vi "Q14070-Z060B bak.vi"() -> ()   [LabVIEW 2013]
uses:
  <vilib>/Utility/file.llb/Read From Spreadsheet File (string).vi
  <vilib>/express/express arith-compare/Formula/XNode/ExpressFormulaBlockNode.xnode
  PCI8622_32.dll
  <vilib>/printing/EasyPrintingControls.llb/contents.ctl
  <vilib>/Utility/NIReport.llb/NI_ReportGenerationCore.lvlib
  <vilib>/printing/EasyPrintingControls.llb/report_type.ctl
  <vilib>/printing/EasyPrinting.llb/Easy Print VI Panel or Documentation (path).vi
  <vilib>/Utility/NIReport.llb/NI_report.lvclass
panel:
  out "最大轴向力标准(N)":dbl=200.0 caption="L+Lmax(mm)" format="%#.3f"
  out "右平均轴向力(N)":dbl caption="L+Lmax(mm)" format="%#.3f"
  out "左平均轴向力(N)":dbl caption="最大位移偏离Lmax(mm)" format="%#.3f"
  in  "确定按钮":bool
  out "员工ID":string
  in  "出支线工步号":dbl
  out "报警提示":string
  in  "报警工步号":dbl
  out "急停":bool
  in  "机械间隙值":dbl
  out "DeviceHandle":u32
  in  "轴向力设定次数":dbl=5.0
  in  "最小间隙(mm)":dbl=0.0005 format="%#.3f"
  out "本备料状态H":bool
  out "本测试状态H":bool
  out "本自动状态H":bool
  out "夹头松开":bool
  out "测头右位":bool
  out "测头左位":bool
  in  "测头气缸右移":bool
  in  "测头气缸左移":bool
  in  "轴向力已做次数":dbl
  out "轴向力及全行程间隙合格":bool
  out "轴向力启动":bool
  out "间隙启动":bool
  out "夹头夹紧位":bool
  in  "夹头松开":bool
  in  "夹头夹紧":bool
  out "找帽扭矩":dbl=1.0 caption="压力传感器" format="%#.2f"
  out "error out":errorcluster
  out "型号数量":i32
  out "error out 4":errorcluster
  in  "间隙设定调整次数":dbl=5.0
  out "读取产品ID":string
  out "本备料状态":bool
  out "本测试状态":bool
  out "本自动状态":bool
  out "FGCS":string
  out "KSJJ":string
  out "Z060BRFID":string
  out "轴向力Y":dbl[](array[numeric])
  out "轴向力X":dbl[](array[numeric])
  out "间隙X数组":dbl[](array[numeric])
  out "间隙Y数组":dbl[](array[numeric])
  out "error out 3":errorcluster caption="错误输出"
  out "rfid工步号":u32
  out "芯片ID":string="201209190001"
  out "rfid完成":bool
  out "rfid触发":bool
  out "本序已做":bool
  in  "回零完成":bool
  in  "电动缸回零":bool
  in  "单点间隙已调试次数":dbl
  in  "需调整角度(度)":dbl
  in  "转向器中心":dbl
  out "扭矩到达":bool
  out "黄灯":bool
  out "红灯":bool
  out "基准位移":dbl caption="压力传感器" format="%#.4f"
  out "上序不合格":bool
  out "单点间隙合格":bool
  out "上序合格":bool
  out "测头机构电机":u32
  out "复位":bool
  in  "型号选择":u16(ring)=1 items=["J709", "J728", "J706"]
  in  "联线按钮":bool
  in  "工步号":u32
  in  "产品ID":string="201209190001"
  out "间隙位移(mm)":dbl caption="压力传感器" format="%#.3f"
  out "齿条推拉力(N)":dbl format="%#.2f"
  out "齿条扭矩(Nm)":dbl format="%#.2f"
  out "通讯状态":bool
  in  "员工ID":string
  out "员工姓名":string
  out "工步提示":string
  out "ADODB._Connection Out 2":refnum<k7>
  out "旋转齿条电机":u32
  out "电动缸电机":u32
  in  "停止":bool
  in  "参数加载":bool
  in  "选项卡控件":T1(tab)
  in  "180°外全行程间隙标准(mm)":dbl=0.1 format="%#.3f"
  out "扭动曲线":cluster{"Y":dbl[], "Y":dbl[]}[](graph) caption="压球涨堵头1"
  out "中间位置间隙":dbl caption="间隙值L(mm)" format="%#.3f"
  in  "中间位置最大间隙标准(mm)":dbl=0.07 format="%#.3f"
  out "右180°外全行程间隙":dbl caption="正向最大间隙L1(mm)" format="%#.3f"
  out "左180°外全行程间隙":dbl caption="正向最大间隙L1(mm)" format="%#.3f"
  out "右180°内全行程间隙":dbl caption="正向最大间隙L1(mm)" format="%#.3f"
  out "左180°内全行程间隙":dbl caption="正向最大间隙L1(mm)" format="%#.3f"
  in  "180°内全行程间隙标准(mm)":dbl=0.07 format="%#.3f"
  in  "找帽OK":bool
  out "左全行程间隙":dbl caption="正向最大间隙L1(mm)" format="%#.3f"
  out "右全行程间隙":dbl caption="正向最大间隙L1(mm)" format="%#.3f"
  out "总圈数最大值":dbl
  out "总圈数标准":dbl
  out "总行程最大值":dbl
  out "总行程标准(mm)":dbl
  out "力波动标准(N)":dbl=60.0 caption="L+Lmax(mm)" format="%#.3f"
  out "平均轴向力标准(N)":dbl=100.0 caption="L+Lmax(mm)" format="%#.3f"
  out "右轴向力波动(N)":dbl caption="L+Lmax(mm)" format="%_5f"
  out "右最大轴向力(N)":dbl caption="L+Lmax(mm)" format="%_5f"
  out "左轴向力波动(N)":dbl caption="最大位移偏离Lmax(mm)" format="%_5f"
  out "左最大轴向力(N)":dbl caption="最大位移偏离Lmax(mm)" format="%_5f"
  out "行程跳动曲线":cluster{"Y":dbl[], "Y":dbl[]}[](graph) caption="压球涨堵头1"
  out "平均轴向力标准(N) max":dbl=200.0 caption="L+Lmax(mm)" format="%#.3f"
  out "总行程":dbl format="%_5g"
  out "总圈数":dbl format="%_1f"
  in  "不合格品":bool
  in  "扭矩停止值":dbl=16.0
  in  "齿条右极限":dbl=-70.0 caption="压力传感器" format="%#.2f"
  in  "齿条左极限":dbl=-262.0 caption="压力传感器" format="%#.2f"
  in  "齿条移动速度":dbl=5.0 caption="压力传感器" format="%#.2f"
  in  "旋转齿条轴找帽转速":dbl=5.0 caption="压力传感器" format="%#.2f"
  in  "测量点扭矩":dbl=4.0 caption="压力传感器" format="%#.2f"
  in  "旋转齿条轴测量转速":dbl caption="压力传感器" format="%#.2f"
  in  "测头机构轴后退位":dbl=30.0 caption="压力传感器" format="%#.2f"
  in  "测头机构轴待检位":dbl caption="压力传感器" format="%#.2f"
  in  "测头机构轴检测位":dbl caption="压力传感器" format="%#.2f"
  in  "测头机构轴移动速度":dbl caption="压力传感器" format="%#.2f"
  in  "机械间隙值":dbl=1.0
  in  "夹头松开":bool
  in  "夹头夹紧":bool
  in  "测头气缸右移":bool
  in  "测头气缸左移":bool
  in  "支线下降":bool
  in  "支线顶升":bool
  in  "出支线":bool
  in  "进支线":bool
  in  "主线下降":bool
  in  "主线顶升":bool
  in  "下阻挡器放行":bool
  in  "上阻挡器放行":bool
  in  "测头机构轴使能":bool
  in  "测头机构轴后退":bool
  in  "测头机构轴前进":bool
  in  "电动缸速度(mm/s)":dbl=10.0 format="%#.3f"
  out "电动缸位置(mm)":dbl=10000.0 format="%#.3f"
  in  "旋转齿条轴速度(°/s)":dbl=10.0 format="%#.3f"
  out "旋转齿条轴位置(°)":dbl=10000.0 format="%#.3f"
  in  "测头机构轴速度(mm/s)":dbl=10.0 format="%#.3f"
  out "测头机构轴位置(mm)":dbl=10000.0 format="%#.3f"
  in  "旋转齿条轴右转":bool
  in  "旋转齿条轴左转":bool
  in  "旋转齿条轴使能":bool
  in  "电动缸后退":bool
  in  "电动缸使能":bool
  in  "电动缸前进":bool
  in  "齿条扭矩比例偏移":dbl=1.0 format="%#.2f"
  in  "齿条扭矩零点偏移":dbl format="%#.2f"
  in  "齿条推拉力比例偏移":dbl=1.0 format="%#.2f"
  in  "齿条推拉力零点偏移":dbl format="%#.2f"
  in  "间隙位移比例偏移":dbl=1.0 format="%#.2f"
  in  "间隙位移零点偏移":dbl format="%#.2f"
  in  "传感器参数保存":bool
  in  "参数修改":bool
  in  "参数查询":bool
  in  "参数浏览表":string[][](table)
  # "芜湖机械转向器装配线"
  # "间隙及轴向力检测"
  # "Q14070机械转向器装配线"
  # "湖北唯思凌科装备制造有限公司 设计开发 (C)2015"
  # "间隙测量结果"
  # "间隙测量判定值"
  # "≤"
  # "≤"
  # "≤"
  # "轴向力测量结果"
  # "轴向力测量标准"
  # "≥"
  # "≤"
  # "≥"
  # "≤"
  # "≤"
  # "≥"
  # "不得大于20NM"
  # "传感器校验区"
  # "关于传感器校验：\n1、传感器校验需要由具备资质的单位或部门进行校验。\n2、具备权限的用户才能够修改传感器校验参数和试验参数。\n3、修改校验参数方法：先将比例偏移置为1，修改零点偏移，使零点值与校验的传感器一致；然后根据增幅调整比例偏移。"
  # "注意：\n具备权限的用户才能够修改传感器校验参数和试验参数！"
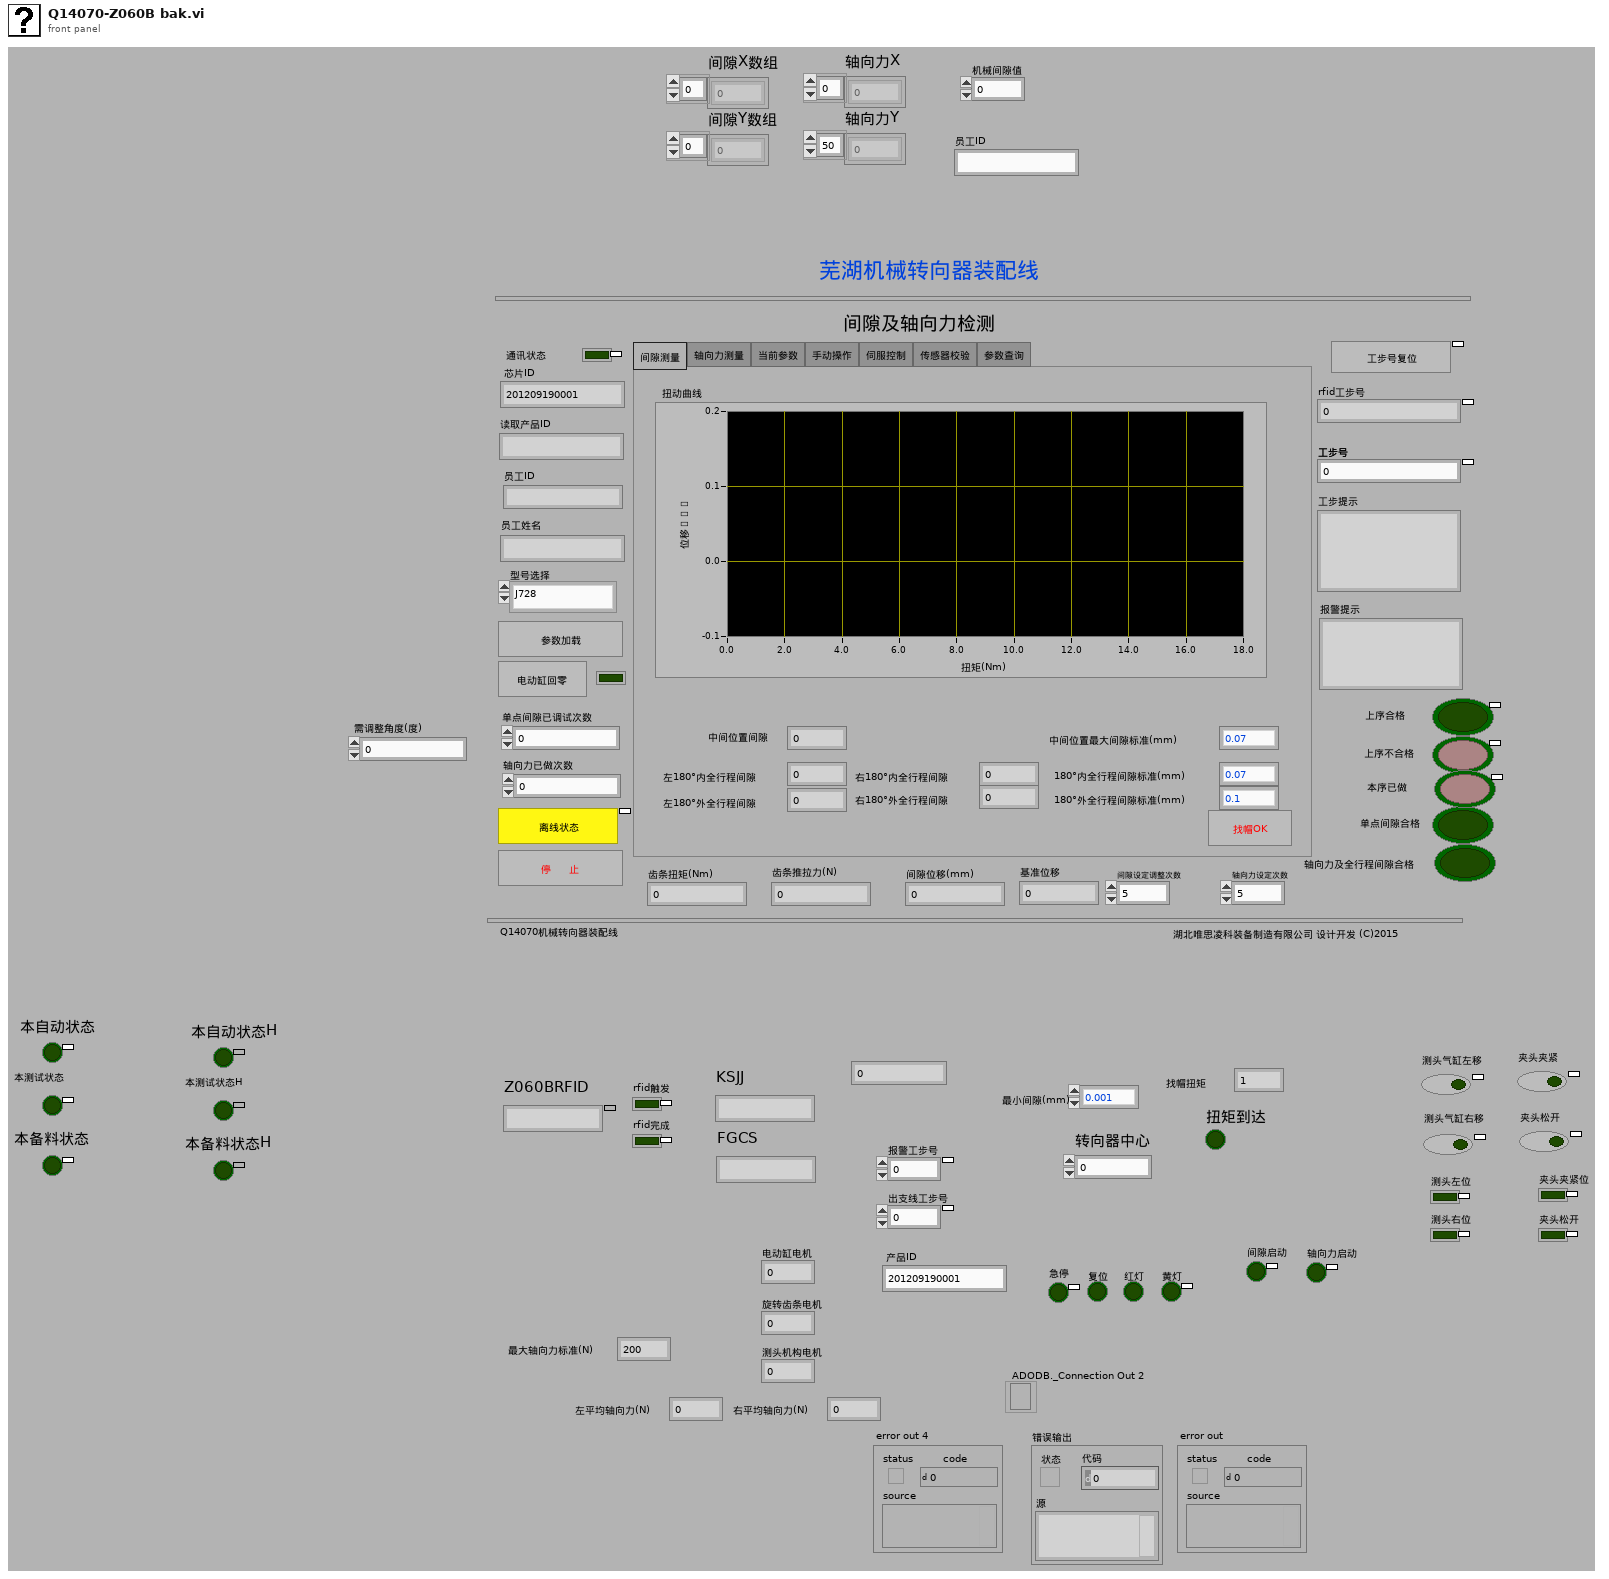
[diagram p1: front panel]
types:
  T1 = enum32{"间隙测量", "轴向力测量", "当前参数", "手动操作", "伺服控制", "传感器校验", "参数查询"}
  T2 = typedef "NI_ReportGenerationCore.lvlib/report_type.ctl" = u16
  T3 = typedef "NI_ReportGenerationCore.lvlib/contents.ctl" = u16
  T4 = typedef "imagedata.ctl" = cluster{"image type":i32, "image depth":i32, "image":u8[], "mask":u8[], "colors":u32[], "Rectangle":cluster{"left":i16, "top":i16, "right":i16, "bottom":i16}}
  T5 = enum8{"Enabled", "Disabled", "Disabled and Grayed Out"}
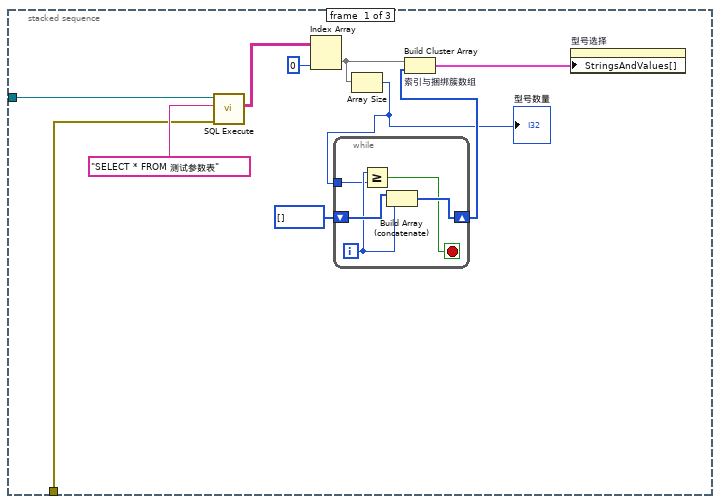
[diagram p4: hidden frame]
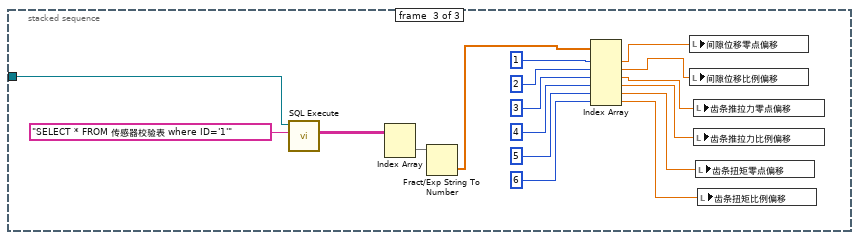
[diagram p5: hidden frame]
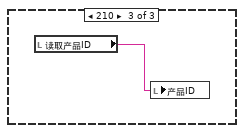
[diagram p7: hidden frame]
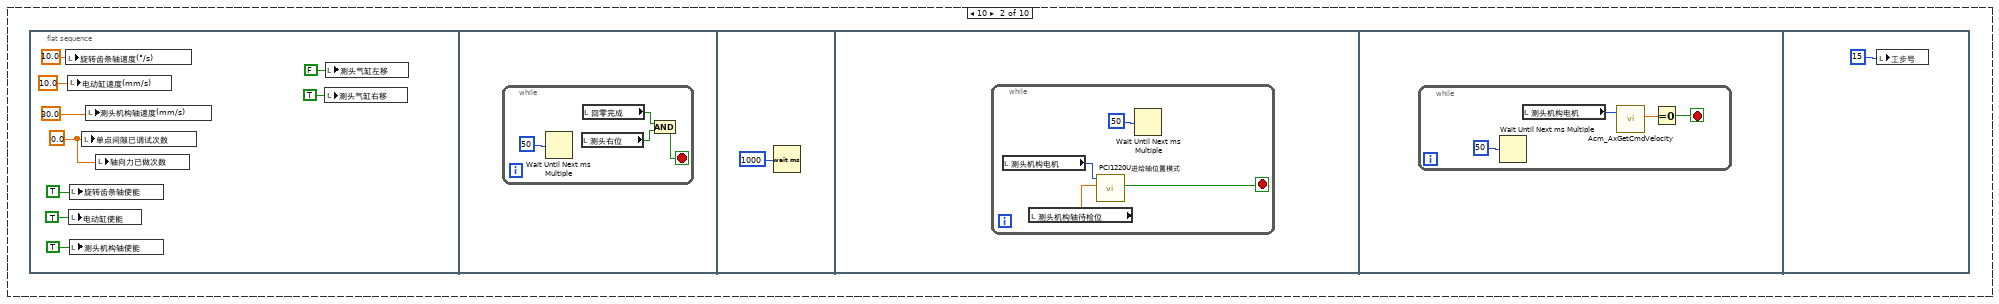
[diagram p9: hidden frame]
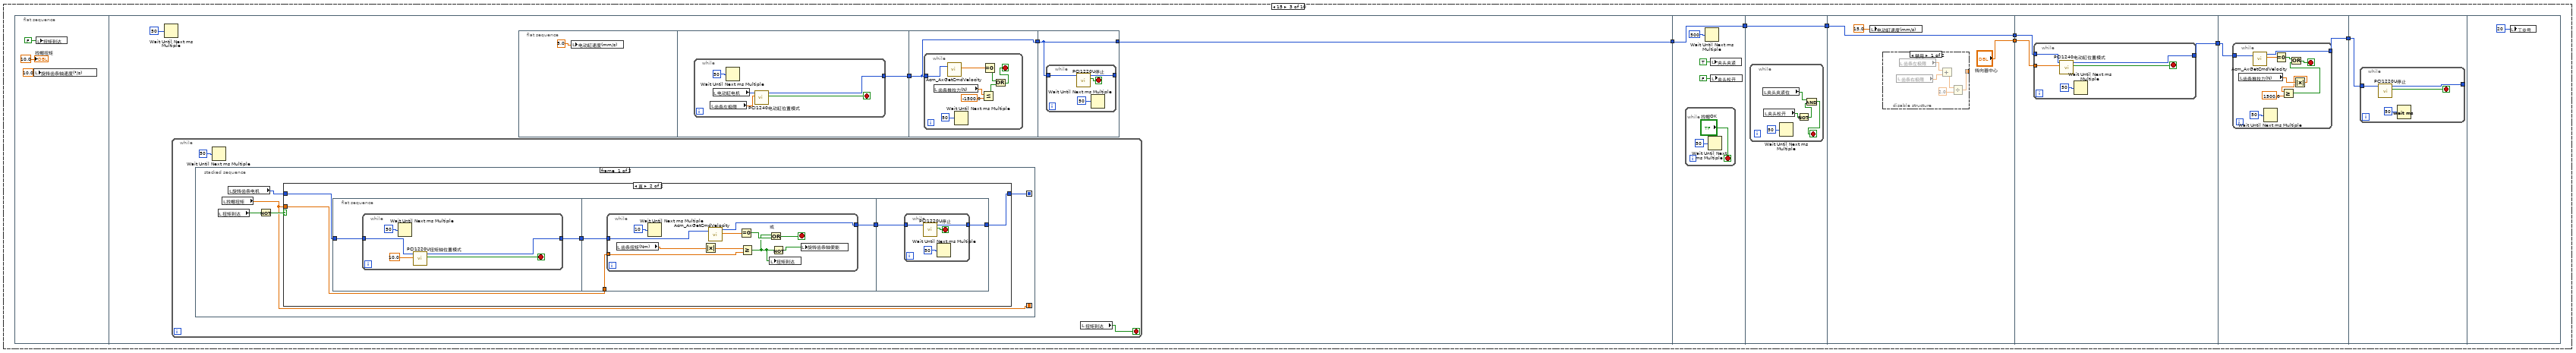
[diagram p10: hidden frame]
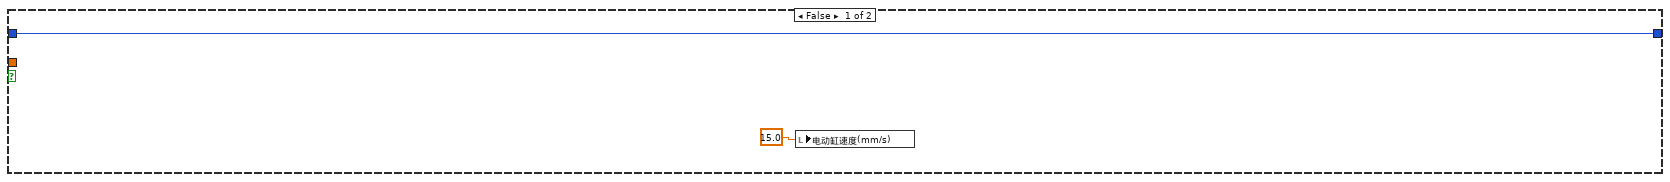
[diagram p11: hidden frame]
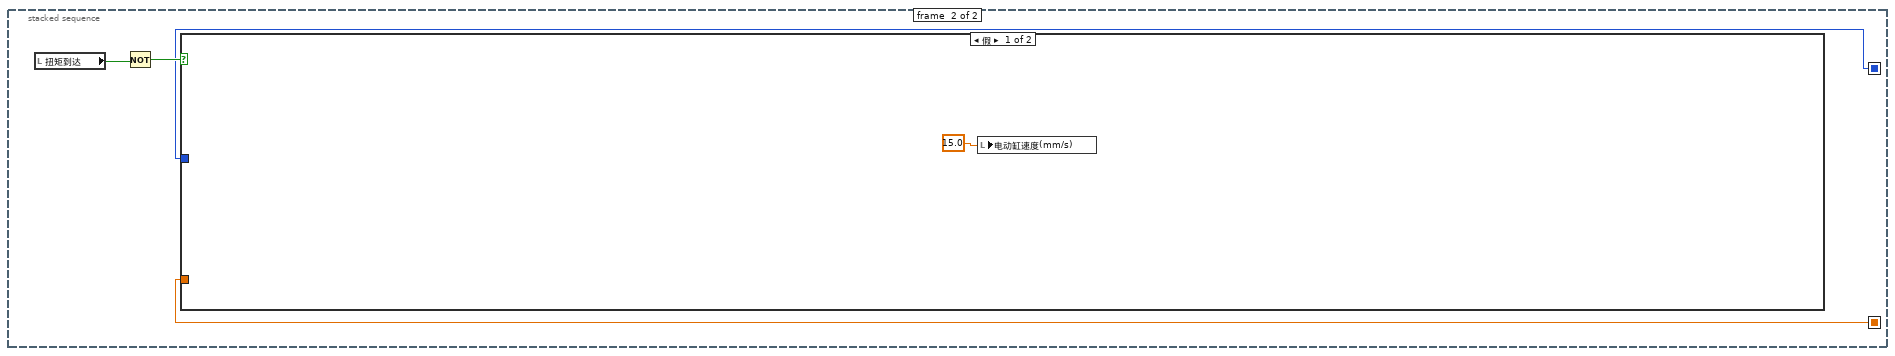
[diagram p12: hidden frame]
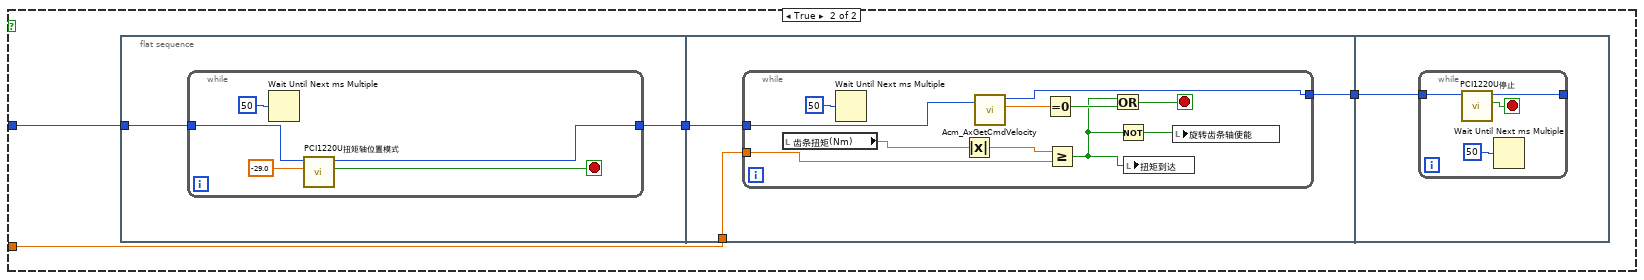
[diagram p13: hidden frame]
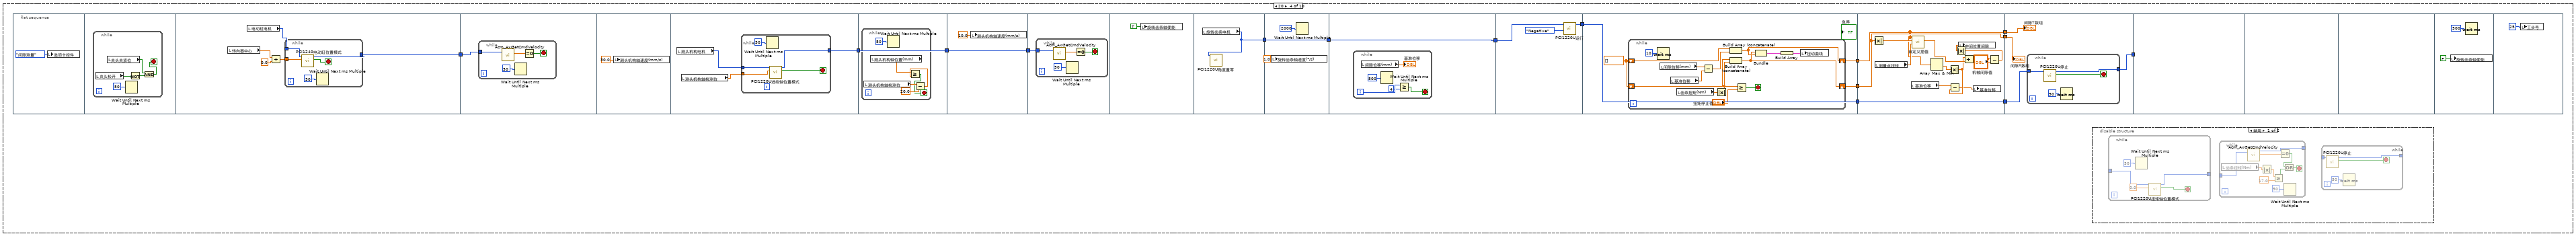
[diagram p15: hidden frame]
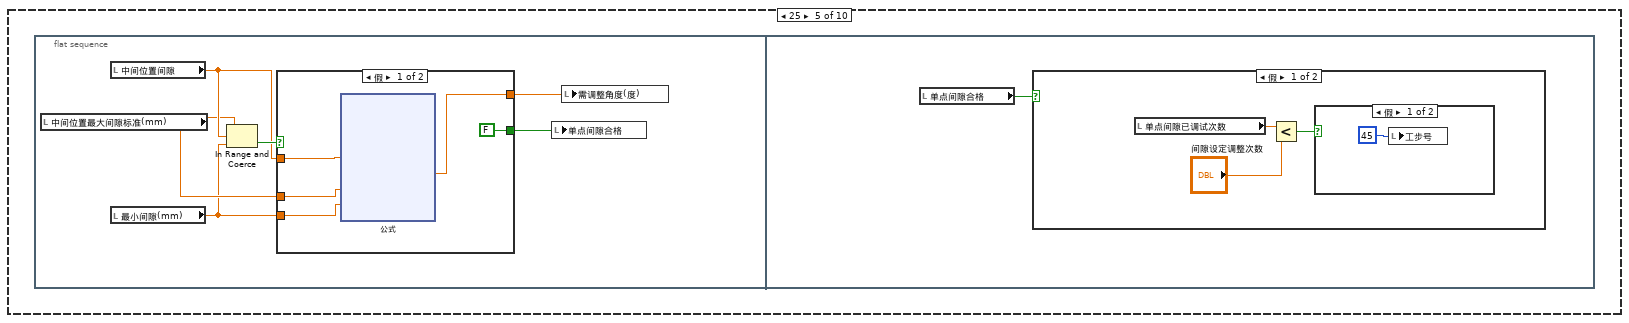
[diagram p17: hidden frame]
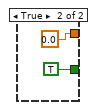
[diagram p18: hidden frame]
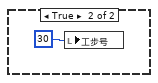
[diagram p19: hidden frame]
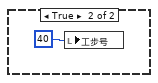
[diagram p20: hidden frame]
diagram:
  n1 = while {
    stop <- w7 stop-if-true
    n2 = local read "工步号"() -> (w5:u32)
    n3 = case shown="40" w5 {
      frame 0, Default {
      }
      frame 10 {
        n4 = flat-sequence {
          frame #0 {
            w8 = 0.0 ("已调试次数")
            n5 = local write "旋转齿条轴速度(°/s)"(10.0 ("旋转齿条轴速度(°/s)")) -> ()
            n6 = local write "电动缸速度(mm/s)"(10.0 ("电动缸速度(mm/s)")) -> ()
            n7 = local write "电动缸使能"(TRUE ("电动缸使能")) -> ()
            n8 = local write "旋转齿条轴使能"(TRUE ("旋转齿条轴使能")) -> ()
            n9 = local write "测头机构轴使能"(TRUE ("调整机构轴使能")) -> ()
            n10 = local write "单点间隙已调试次数"(w8) -> ()
            n11 = local write "测头机构轴速度(mm/s)"(30.0 ("调整机构轴速度(mm/s)")) -> ()
            n12 = local write "轴向力已做次数"(w8) -> ()
            n13 = local write "测头气缸右移"(TRUE ("测头气缸右移")) -> ()
            n14 = local write "测头气缸左移"(FALSE ("测头气缸左移")) -> ()
          }
          frame #1 {
            n15 = while {
              stop <- w17 stop-if-true
              n16 = Wait Until Next ms Multiple(millisecond multiple=u32 50 ("毫秒倍数")) -> ()  [unwired: 1 out]
              n17 = local read "测头右位"() -> (w18:bool)
              n18 = local read "回零完成"() -> (w19:bool)
              n19 = And(x=w19, y=w18) -> (x .and. y?=w17:bool)
            }
          }
          frame #2 {
            n20 = Wait (ms)(milliseconds to wait=u32 1000 ("等待时间（毫秒）")) -> ()  [unwired: 1 out]
          }
          frame #3 {
            n21 = while {
              stop <- w25 stop-if-true
              n22 = local read "测头机构电机"() -> (w23:u32)
              n23 = local read "测头机构轴待检位"() -> (w22:dbl)
              n24 = call "PCI1220U进给轴位置模式.vi"("Distance"=w22, "AxisHandle IN"=w23) -> ("AbsSuccess"=w25:bool)  [unwired: 8 in, 1 out]
              n25 = Wait Until Next ms Multiple(millisecond multiple=u32 50 ("毫秒倍数")) -> ()  [unwired: 1 out]
            }
          }
          frame #4 {
            n26 = while {
              stop <- w28 stop-if-true
              n27 = Wait Until Next ms Multiple(millisecond multiple=u32 50 ("毫秒倍数")) -> ()  [unwired: 1 out]
              n28 = local read "测头机构电机"() -> (w26:u32)
              n29 = call <userlib>:"Acm_AxGetCmdVelocity.vi"("AxisHandle"=w26) -> ("Velocity"=w29:dbl)  [unwired: 1 in, 3 out]
              n30 = Equal To 0?(x=w29) -> (x = 0?=w28:bool)
            }
          }
          frame #5 {
            n31 = local write "工步号"(u32 15 ("工步号")) -> ()
          }
        }
      }
      frame 15 {
        n32 = flat-sequence {
          tunnel: [w42] -> w34
          tunnel: w34 -> [w144]
          tunnel: [w144] -> w32
          tunnel: w32 -> [w148]
          tunnel: [w148] -> w31
          tunnel: [w155] -> w37
          tunnel: ["转向器中心"] -> w36
          tunnel: w31 -> [w155]
          tunnel: w37 -> [w164]
          tunnel: w36 -> [w163]
          tunnel: [w162] -> w35
          tunnel: w35 -> [w171]
          tunnel: [w170] -> w33
          tunnel: w33 -> [w182]
          frame #0 {
            n33 = local write "旋转齿条轴速度(°/s)"(10.0 ("旋转齿条轴速度(°/s)")) -> ()
            n34 = local write "扭矩到达"(FALSE ("扭矩到达")) -> ()
            "找帽扭矩" <- 10.0 ("找帽扭矩")
          }
          frame #1 {
            n35 = Wait Until Next ms Multiple(millisecond multiple=u32 50 ("毫秒倍数")) -> ()  [unwired: 1 out]
            n36 = while {
              stop <- w45 stop-if-true
              n37 = stacked-sequence {
                seq-local: [w47 _] -> [_ w88]
                seq-local: [w51 _] -> [_ w87]
                frame #0 {
                  n38 = local read "扭矩到达"() -> (w49:bool)
                  n39 = local read "找帽扭矩"() -> (w47:dbl)
                  n40 = local read "旋转齿条电机"() -> (w48:u32)
                  n41 = Not(x=w49) -> (.not. x?=w50:bool)
                  n42 = case shown="真" w50 {
                    tunnel: [w53 w54] -> w51
                    tunnel: w48 -> [w53 w58]
                    tunnel: w47 -> [_ w56]
                    frame False {
                      n43 = local write "电动缸速度(mm/s)"(15.0 ("电动缸速度(mm/s)")) -> ()
                    }
                    frame True {
                      n44 = flat-sequence {
                        tunnel: w58 -> [w60]
                        tunnel: [w59] -> w57
                        tunnel: w57 -> [w68]
                        tunnel: w56 -> [w67]
                        tunnel: [w66] -> w55
                        tunnel: w55 -> [w81]
                        tunnel: [w80] -> w54
                        frame #0 {
                          n45 = while {
                            tunnel: [w64] -> w59
                            tunnel: w60 -> [w61]
                            stop <- w63 stop-if-true
                            n46 = Wait Until Next ms Multiple(millisecond multiple=u32 50 ("毫秒倍数")) -> ()  [unwired: 1 out]
                            n47 = call "PCI1220U扭矩轴位置模式.vi"("Distance"=10.0, "AxisHandle IN"=w61) -> ("AbsSuccess"=w63:bool, "AxisHandle OUT"=w64:u32)  [unwired: 8 in]
                          }
                        }
                        frame #1 {
                          n48 = while {
                            tunnel: w68 -> [w78]
                            tunnel: w67 -> [w73]
                            tunnel: [w72] -> w66
                            stop <- w74 stop-if-true
                            n49 = local read "齿条扭矩(Nm)"() -> (w71:dbl)
                            n50 = Wait Until Next ms Multiple(millisecond multiple=u32 10 ("毫秒倍数")) -> ()  [unwired: 1 out]
                            n51 = Absolute Value(x=w71) -> (abs(x)=w76:dbl)
                            n52 = call <userlib>:"Acm_AxGetCmdVelocity.vi"("AxisHandle"=w78) -> ("Velocity"=w77:dbl, "AxisHandle"=w72:u32)  [unwired: 1 in, 2 out]
                            n53 = Equal To 0?(x=w77) -> (x = 0?=w75:bool)
                            n54 = Greater Or Equal?(x=w76, y=w73) -> (x >= y?=w70:bool)
                            n55 = Or "或"(x=w70, y=w75) -> (x .or. y?=w74:bool)
                            n56 = local write "扭矩到达"(w70) -> ()
                            n57 = Not(x=w70) -> (.not. x?=w69:bool)
                            n58 = local write "旋转齿条轴使能"(w69) -> ()
                          }
                        }
                        frame #2 {
                          n59 = while {
                            tunnel: w81 -> [w85]
                            tunnel: [w82] -> w80
                            stop <- w84 stop-if-true
                            n60 = call "PCI1220U停止.vi"("AxisHandle IN"=w85) -> ("完成"=w84:bool, "AxisHandle OUT"=w82:u32)  [unwired: 9 in]
                            n61 = Wait Until Next ms Multiple(millisecond multiple=u32 50 ("毫秒倍数")) -> ()  [unwired: 1 out]
                          }
                        }
                      }
                    }
                  }
                }
                frame #1 {
                  n62 = local read "扭矩到达"() -> (w86:bool)
                  n63 = Not(x=w86) -> (.not. x?=w89:bool)
                  n64 = case shown="假" w89 {
                    tunnel: w87 -> [_ w94]
                    tunnel: w88 -> [_ w92]
                    frame False {
                      n65 = local write "电动缸速度(mm/s)"(15.0 ("电动缸速度(mm/s)")) -> ()
                    }
                    frame True {
                      n66 = flat-sequence {
                        tunnel: w94 -> [w95]
                        tunnel: [w96] -> w93
                        tunnel: w93 -> [w104]
                        tunnel: w92 -> [w103]
                        tunnel: [w102] -> w91
                        tunnel: w91 -> [w116]
                        frame #0 {
                          n67 = while {
                            tunnel: [w100] -> w96
                            tunnel: w95 -> [w97]
                            stop <- w99 stop-if-true
                            n68 = Wait Until Next ms Multiple(millisecond multiple=u32 50 ("毫秒倍数")) -> ()  [unwired: 1 out]
                            n69 = call "PCI1220U扭矩轴位置模式.vi"("Distance"=-29.0, "AxisHandle IN"=w97) -> ("AbsSuccess"=w99:bool, "AxisHandle OUT"=w100:u32)  [unwired: 8 in]
                          }
                        }
                        frame #1 {
                          n70 = while {
                            tunnel: w104 -> [w114]
                            tunnel: [w109] -> w102
                            tunnel: w103 -> [w108]
                            stop <- w110 stop-if-true
                            n71 = local read "齿条扭矩(Nm)"() -> (w107:dbl)
                            n72 = Wait Until Next ms Multiple(millisecond multiple=u32 50 ("毫秒倍数")) -> ()  [unwired: 1 out]
                            n73 = Absolute Value(x=w107) -> (abs(x)=w112:dbl)
                            n74 = call <userlib>:"Acm_AxGetCmdVelocity.vi"("AxisHandle"=w114) -> ("Velocity"=w113:dbl, "AxisHandle"=w109:u32)  [unwired: 1 in, 2 out]
                            n75 = Equal To 0?(x=w113) -> (x = 0?=w111:bool)
                            n76 = Greater Or Equal?(x=w112, y=w108) -> (x >= y?=w105:bool)
                            n77 = Or(x=w105, y=w111) -> (x .or. y?=w110:bool)
                            n78 = Not(x=w105) -> (.not. x?=w106:bool)
                            n79 = local write "扭矩到达"(w105) -> ()
                            n80 = local write "旋转齿条轴使能"(w106) -> ()
                          }
                        }
                        frame #2 {
                          n81 = while {
                            tunnel: w116 -> [w120]
                            tunnel: [w117] -> _
                            stop <- w119 stop-if-true
                            n82 = call "PCI1220U停止.vi"("AxisHandle IN"=w120) -> ("完成"=w119:bool, "AxisHandle OUT"=w117:u32)  [unwired: 9 in]
                            n83 = Wait Until Next ms Multiple(millisecond multiple=u32 50 ("毫秒倍数")) -> ()  [unwired: 1 out]
                          }
                        }
                      }
                    }
                  }
                }
              }
              n84 = Wait Until Next ms Multiple(millisecond multiple=u32 50 ("毫秒倍数")) -> ()  [unwired: 1 out]
              n85 = local read "扭矩到达"() -> (w45:bool)
            }
            n86 = flat-sequence {
              tunnel: [w122] -> w44
              tunnel: w44 -> [w128]
              tunnel: [w128] -> w41
              tunnel: [w137] -> w42
              tunnel: w41 -> [w137]
              frame #0 {
                n87 = local write "电动缸速度(mm/s)"(5.0 ("电动缸速度(mm/s)")) -> ()
              }
              frame #1 {
                n88 = while {
                  tunnel: [w126] -> w122
                  stop <- w125 stop-if-true
                  n89 = local read "齿条左极限"() -> (w123:dbl)
                  n90 = local read "电动缸电机"() -> (w127:u32)
                  n91 = Wait Until Next ms Multiple(millisecond multiple=u32 50 ("毫秒倍数")) -> ()  [unwired: 1 out]
                  n92 = call "PCI1240电动缸位置模式 .vi"("Distance"=w123, "AxisHandle IN"=w127) -> ("AbsSuccess"=w125:bool, "AxisHandle OUT"=w126:u32)  [unwired: 8 in]
                }
              }
              frame #2 {
                n93 = while {
                  tunnel: w128 -> [w135]
                  stop <- w132 stop-if-true
                  n94 = local read "齿条推拉力(N)"() -> (w131:dbl)
                  n95 = call <userlib>:"Acm_AxGetCmdVelocity.vi"("AxisHandle"=w135) -> ("Velocity"=w136:dbl)  [unwired: 1 in, 3 out]
                  n96 = Wait Until Next ms Multiple(millisecond multiple=u32 50 ("毫秒倍数")) -> ()  [unwired: 1 out]
                  n97 = Less Or Equal?(x=w131, y=-1500.0) -> (x <= y?=w129:bool)
                  n98 = Equal To 0?(x=w136) -> (x = 0?=w133:bool)
                  n99 = Or(x=w133, y=w129) -> (x .or. y?=w132:bool)
                }
              }
              frame #3 {
                n100 = while {
                  tunnel: w137 -> [w141]
                  tunnel: [w138] -> _
                  stop <- w140 stop-if-true
                  n101 = call "PCI1220U停止.vi"("AxisHandle IN"=w141) -> ("完成"=w140:bool, "AxisHandle OUT"=w138:u32)  [unwired: 9 in]
                  n102 = Wait Until Next ms Multiple(millisecond multiple=u32 50 ("毫秒倍数")) -> ()  [unwired: 1 out]
                }
              }
            }
          }
          frame #2 {
            n103 = while {
              stop <- "找帽OK" stop-if-true
              n104 = Wait Until Next ms Multiple(millisecond multiple=u32 50 ("毫秒倍数")) -> ()  [unwired: 1 out]
            }
            n105 = Wait Until Next ms Multiple(millisecond multiple=u32 500 ("毫秒倍数")) -> ()  [unwired: 1 out]
            n106 = local write "夹头夹紧"(TRUE ("夹头夹紧")) -> ()
            n107 = local write "夹头松开"(FALSE ("夹头松开")) -> ()
          }
          frame #3 {
            n108 = while {
              stop <- w150 stop-if-true
              n109 = local read "夹头夹紧位"() -> (w151:bool)
              n110 = local read "夹头松开"() -> (w153:bool)
              n111 = Wait Until Next ms Multiple(millisecond multiple=u32 50 ("毫秒倍数")) -> ()  [unwired: 1 out]
              n112 = Not(x=w153) -> (.not. x?=w152:bool)
              n113 = And(x=w151, y=w152) -> (x .and. y?=w150:bool)
            }
          }
          frame #4 {
            n114 = local write "电动缸速度(mm/s)"(15.0 ("电动缸轴移动速度")) -> ()
            n115 = disable-structure shown="禁用" {
              disable-tunnel: [w157 _] -> _
              frame Disabled {
                n116 = local read "齿条右极限"() -> (w160:dbl)
                n117 = local read "齿条左极限"() -> (w161:dbl)
                n118 = Add(x=w161, y=w160) -> (x+y=w159:dbl)
                n119 = Divide(x=w159, y=2.0) -> (x/y=w157:dbl)
              }
              frame Enabled {
              }
            }
          }
          frame #5 {
            n120 = while {
              tunnel: w164 -> [w169]
              tunnel: w163 -> [w168]
              tunnel: [w165] -> w162
              stop <- w167 stop-if-true
              n121 = call "PCI1240电动缸位置模式 .vi"("Distance"=w168, "AxisHandle IN"=w169) -> ("AbsSuccess"=w167:bool, "AxisHandle OUT"=w165:u32)  [unwired: 8 in]
              n122 = Wait Until Next ms Multiple(millisecond multiple=u32 50 ("毫秒倍数")) -> ()  [unwired: 1 out]
            }
          }
          frame #6 {
            n123 = while {
              tunnel: w171 -> [w181]
              tunnel: [w172] -> w170
              stop <- w173 stop-if-true
              n124 = local read "齿条推拉力(N)"() -> (w178:dbl)
              n125 = call <userlib>:"Acm_AxGetCmdVelocity.vi"("AxisHandle"=w181) -> ("Velocity"=w180:dbl, "AxisHandle"=w172:u32)  [unwired: 1 in, 2 out]
              n126 = Wait Until Next ms Multiple(millisecond multiple=u32 50 ("毫秒倍数")) -> ()  [unwired: 1 out]
              n127 = Equal To 0?(x=w180) -> (x = 0?=w175:bool)
              n128 = Absolute Value(x=w178) -> (abs(x)=w177:dbl)
              n129 = Greater Or Equal?(x=w177, y=1500.0) -> (x >= y?=w174:bool)
              n130 = Or(x=w175, y=w174) -> (x .or. y?=w173:bool)
            }
          }
          frame #7 {
            n131 = while {
              tunnel: w182 -> [w186]
              tunnel: [w185] -> _
              stop <- w184 stop-if-true
              n132 = call "PCI1220U停止.vi"("AxisHandle IN"=w186) -> ("完成"=w184:bool, "AxisHandle OUT"=w185:u32)  [unwired: 9 in]
              n133 = Wait (ms)(milliseconds to wait=u32 50 ("毫秒倍数")) -> ()  [unwired: 1 out]
            }
          }
          frame #8 {
            n134 = local write "工步号"(u32 20 ("工步号")) -> ()
          }
        }
      }
      frame 20 {
        n135 = flat-sequence {
          tunnel: [w232] -> w194
          tunnel: w194 -> [w238]
          tunnel: [w245] -> w190
          tunnel: w190 -> [w252]
          tunnel: [w252] -> w189
          tunnel: w189 -> [w260]
          tunnel: [w260] -> w188
          tunnel: w188 -> [w261]
          tunnel: [w267] -> w192
          tunnel: [w269] -> w193
          tunnel: w192 -> [w269]
          tunnel: [w271] -> w199
          tunnel: w193 -> [w271]
          tunnel: w199 -> [w278]
          tunnel: [w277] -> w198
          tunnel: [w282] -> w197
          tunnel: [w281] -> w196
          tunnel: w198 -> [w280]
          tunnel: [w280] -> w195
          tunnel: [w311] -> w202
          tunnel: [w308] -> w201
          tunnel: w197 -> [w308]
          tunnel: [w307] -> w200
          tunnel: w196 -> [w307]
          tunnel: w195 -> [w311]
          tunnel: w202 -> [w315]
          tunnel: [w314] -> w191
          tunnel: w201 -> [w312]
          tunnel: w200 -> [w313]
          tunnel: w191 -> [_]
          frame #0 {
            n136 = local write "选项卡控件"(T1."间隙测量" ("选项卡控件")) -> ()
          }
          frame #1 {
            n137 = while {
              stop <- w223 stop-if-true
              n138 = local read "夹头松开"() -> (w225:bool)
              n139 = local read "夹头夹紧位"() -> (w224:bool)
              n140 = Wait Until Next ms Multiple(millisecond multiple=u32 50 ("毫秒倍数")) -> ()  [unwired: 1 out]
              n141 = Not(x=w225) -> (.not. x?=w226:bool)
              n142 = And(x=w224, y=w226) -> (x .and. y?=w223:bool)
            }
          }
          frame #2 {
            n143 = local read "转向器中心"() -> (w228:dbl)
            n144 = local read "电动缸电机"() -> (w231:u32)
            n145 = Add(x=w228, y=0.0) -> (x+y=w230:dbl)
            n146 = while {
              tunnel: w231 -> [w237]
              tunnel: w230 -> [w236]
              tunnel: [w233] -> w232
              stop <- w235 stop-if-true
              n147 = call "PCI1240电动缸位置模式 .vi"("Distance"=w236, "AxisHandle IN"=w237) -> ("AbsSuccess"=w235:bool, "AxisHandle OUT"=w233:u32)  [unwired: 8 in]
              n148 = Wait Until Next ms Multiple(millisecond multiple=u32 50 ("毫秒倍数")) -> ()  [unwired: 1 out]
            }
          }
          frame #3 {
            n149 = while {
              tunnel: w238 -> [w242]
              stop <- w240 stop-if-true
              n150 = call <userlib>:"Acm_AxGetCmdVelocity.vi"("AxisHandle"=w242) -> ("Velocity"=w241:dbl)  [unwired: 1 in, 3 out]
              n151 = Wait Until Next ms Multiple(millisecond multiple=u32 50 ("毫秒倍数")) -> ()  [unwired: 1 out]
              n152 = Equal To 0?(x=w241) -> (x = 0?=w240:bool)
            }
          }
          frame #4 {
            n153 = local write "测头机构轴速度(mm/s)"(30.0 ("测头机构轴速度(mm/s)")) -> ()
          }
          frame #5 {
            n154 = local read "测头机构电机"() -> (w246:u32)
            n155 = local read "测头机构轴检测位"() -> (w244:dbl)
            n156 = while {
              tunnel: w246 -> [w249]
              tunnel: w244 -> [w248]
              tunnel: [w247] -> w245
              stop <- w251 stop-if-true
              n157 = Wait Until Next ms Multiple(millisecond multiple=u32 50 ("毫秒倍数")) -> ()  [unwired: 1 out]
              n158 = call "PCI1220U进给轴位置模式.vi"("Distance"=w248, "AxisHandle IN"=w249) -> ("AbsSuccess"=w251:bool, "AxisHandle OUT"=w247:u32)  [unwired: 8 in]
            }
          }
          frame #6 {
            n159 = while {
              stop <- w255 stop-if-true
              n160 = local read "测头机构轴检测位"() -> (w257:dbl)
              n161 = local read "测头机构轴位置(mm)"() -> (w254:dbl)
              n162 = Wait Until Next ms Multiple(millisecond multiple=u32 50 ("毫秒倍数")) -> ()  [unwired: 1 out]
              n163 = Subtract(x=w257, y=20.0) -> (x-y=w253:dbl)
              n164 = Greater Or Equal?(x=w254, y=w253) -> (x >= y?=w255:bool)
            }
          }
          frame #7 {
            n165 = local write "测头机构轴速度(mm/s)"(10.0 ("测头机构轴速度(mm/s)")) -> ()
          }
          frame #8 {
            n166 = while {
              tunnel: w261 -> [w265]
              stop <- w263 stop-if-true
              n167 = call <userlib>:"Acm_AxGetCmdVelocity.vi"("AxisHandle"=w265) -> ("Velocity"=w264:dbl)  [unwired: 1 in, 3 out]
              n168 = Wait Until Next ms Multiple(millisecond multiple=u32 50 ("毫秒倍数")) -> ()  [unwired: 1 out]
              n169 = Equal To 0?(x=w264) -> (x = 0?=w263:bool)
            }
          }
          frame #9 {
            n170 = local write "旋转齿条轴使能"(TRUE ("旋转齿条轴使能")) -> ()
          }
          frame #10 {
            n171 = local read "旋转齿条电机"() -> (w267:u32)
            n172 = call "PCI1220U角度置零.vi"("AxisHandle IN"=w267) -> ()  [unwired: 10 in, 1 out]
          }
          frame #11 {
            n173 = local write "旋转齿条轴速度(°/s)"(1.0 ("旋转齿条轴速度(°/s)")) -> ()
            n174 = Wait Until Next ms Multiple(millisecond multiple=u32 2000 ("毫秒倍数")) -> ()  [unwired: 1 out]
          }
          frame #12 {
            n175 = while {
              i -> [w274]
              stop <- w272 stop-if-true
              n176 = local read "间隙位移(mm)"() -> (→"基准位移":dbl)
              n177 = Wait Until Next ms Multiple(millisecond multiple=u32 500 ("毫秒倍数")) -> ()  [unwired: 1 out]
              n178 = Greater Or Equal?(x=w274, y=4) -> (x >= y?=w272:bool)
            }
          }
          frame #13 {
            n179 = call "PCI1220U运行.vi"("方向"=enum32{"Negative", "Positive"}."Negative" ("Direction"), "AxisHandle IN"=w278) -> ("AxisHandle OUT"=w277:u32)  [unwired: 9 in]
          }
          frame #14 {
            w283 = dbl[] []
            n180 = while {
              shift-right: [w294] -> w282
              shift-left: w283 -> [w296]
              shift-right: [w293] -> w281
              shift-left: w283 -> [w295]
              stop <- w286 stop-if-true
              n181 = Wait (ms)(milliseconds to wait=u32 10 ("毫秒倍数")) -> ()  [unwired: 1 out]
              n182 = local read "间隙位移(mm)"() -> (w289:dbl)
              n183 = local read "基准位移"() -> (w287:dbl)
              n184 = local read "齿条扭矩(Nm)"() -> (w290:dbl)
              n185 = Subtract(x=w289, y=w287) -> (x-y=w288:dbl)
              n186 = Absolute Value(x=w290) -> (abs(x)=w285:dbl)
              n187 = Build Array (concatenate) ("创建数组")(w295, w288) -> (w293:dbl[])
              n188 = Build Array (concatenate) ("创建数组")(w296, w285) -> (w294:dbl[])
              n189 = Greater Or Equal?(x=w285, y="扭矩停止值") -> (x >= y?=w286:bool)
              n190 = Bundle ("捆绑")(w294, w293) -> (w291:cluster{dbl[], dbl[]})  [unwired: 1 in]
              n191 = Build Array ("创建数组")(w291) -> (w292:cluster{dbl[], dbl[]}[])
              n192 = local write "扭动曲线"(w292) -> ()
            }
          }
          frame #15 {
            n193 = Absolute Value(x=w308) -> (abs(x)=w309:dbl[])
            n194 = local read "测量点扭矩"() -> (w310:dbl)
            n195 = local read "基准位移"() -> (w304:dbl)
            n196 = call "自定义插值.vi"("压力"=w310, "扭矩数组"=w309, "位移数组"=w307) -> ("扭矩值"=w305:dbl)  [unwired: 8 in]
            n197 = Array Max & Min(array=w307) -> (min value=w306:dbl)  [unwired: 3 out]
            n198 = Absolute Value(x=w306) -> (abs(x)=w303:dbl)
            n199 = Subtract(x=w304, y=w303) -> (x-y=w302:dbl)
            n200 = Add(x=w303, y=w305) -> (x+y=w300:dbl)
            n201 = local write "基准位移"(w302) -> ()
            n202 = Subtract(x=w300, y="机械间隙值") -> (x-y=w301:dbl)
            n203 = Absolute Value(x=w301) -> (abs(x)=w298:dbl)
            n204 = local write "中间位置间隙"(w298) -> ()
          }
          frame #16 {
            n205 = while {
              tunnel: w315 -> [w319]
              tunnel: [w318] -> w314
              stop <- w317 stop-if-true
              n206 = call "PCI1220U停止.vi"("AxisHandle IN"=w319) -> ("完成"=w317:bool, "AxisHandle OUT"=w318:u32)  [unwired: 9 in]
              n207 = Wait (ms)(milliseconds to wait=u32 50 ("毫秒倍数")) -> ()  [unwired: 1 out]
            }
            "间隙Y数组" <- w313
            "间隙X数组" <- w312
          }
          frame #17 {
          }
          frame #18 {
          }
          frame #19 {
          }
          frame #20 {
            n208 = local write "旋转齿条轴使能"(FALSE ("旋转齿条轴使能")) -> ()
            n209 = Wait (ms)(milliseconds to wait=u32 500 ("毫秒倍数")) -> ()  [unwired: 1 out]
          }
          frame #21 {
            n210 = local write "工步号"(u32 25 ("工步号")) -> ()
          }
        }
        n211 = disable-structure shown="禁用" {
          frame Disabled {
            n212 = while {
              tunnel: [w221] -> _
              tunnel: _ -> [w219]
              stop <- w220 stop-if-true
              n213 = Wait Until Next ms Multiple(millisecond multiple=u32 50 ("毫秒倍数")) -> ()  [unwired: 1 out]
              n214 = call "PCI1220U扭矩轴位置模式.vi"("Distance"=0.0, "AxisHandle IN"=w219) -> ("AbsSuccess"=w220:bool, "AxisHandle OUT"=w221:u32)  [unwired: 8 in]
            }
            n215 = while {
              tunnel: _ -> [w215]
              tunnel: [w207] -> _
              stop <- w208 stop-if-true
              n216 = local read "齿条扭矩(Nm)"() -> (w211:dbl)
              n217 = call <userlib>:"Acm_AxGetCmdVelocity.vi"("AxisHandle"=w215) -> ("Velocity"=w216:dbl, "AxisHandle"=w207:u32)  [unwired: 1 in, 2 out]
              n218 = Absolute Value(x=w211) -> (abs(x)=w212:dbl)
              n219 = Greater Or Equal?(x=w212, y=17.0) -> (x >= y?=w209:bool)
              n220 = Equal To 0?(x=w216) -> (x = 0?=w210:bool)
              n221 = Or(x=w210, y=w209) -> (x .or. y?=w208:bool)
              n222 = Wait Until Next ms Multiple(millisecond multiple=u32 50 ("毫秒倍数")) -> ()  [unwired: 1 out]
            }
            n223 = while {
              tunnel: _ -> [w206]
              tunnel: [w205] -> _
              stop <- w204 stop-if-true
              n224 = call "PCI1220U停止.vi"("AxisHandle IN"=w206) -> ("完成"=w204:bool, "AxisHandle OUT"=w205:u32)  [unwired: 9 in]
              n225 = Wait (ms)(milliseconds to wait=u32 50 ("毫秒倍数")) -> ()  [unwired: 1 out]
            }
          }
          frame Enabled {
          }
        }
      }
      frame 25 {
        n226 = flat-sequence {
          frame #0 {
            n227 = local read "中间位置最大间隙标准(mm)"() -> (w324:dbl)
            n228 = local read "中间位置间隙"() -> (w325:dbl)
            n229 = local read "最小间隙(mm)"() -> (w323:dbl)
            n230 = In Range and Coerce(upper limit=w324, x=w325, lower limit=w323) -> (In Range?=w328:bool)  [unwired: 1 out]
            n231 = case shown="假" w328 {
              tunnel: [FALSE ("本序合格") TRUE ("本序合格")] -> w327
              tunnel: [w333 0.0 ("需调整角度(度)")] -> w326
              tunnel: w325 -> [w331 _]
              tunnel: w324 -> [w330 _]
              tunnel: w323 -> [w329 _]
              frame False {
                n232 = xnode "公式"("X"=w331, "Xmax"=w330, "Xmin"=w329) -> ("结果"=w333:dbl)  [unwired: 1 in, 1 out]
              }
              frame True {
              }
            }
            n233 = local write "单点间隙合格"(w327) -> ()
            n234 = local write "需调整角度(度)"(w326) -> ()
          }
          frame #1 {
            n235 = local read "单点间隙合格"() -> (w348:bool)
            n236 = case shown="假" w348 {
              frame False {
                n237 = local read "单点间隙已调试次数"() -> (w351:dbl)
                n238 = Less?(x=w351, y="间隙设定调整次数") -> (x < y?=w350:bool)
                n239 = case shown="假" w350 {
                  frame False {
                    n240 = local write "工步号"(u32 45 ("变更工步号")) -> ()
                  }
                  frame True {
                    n241 = local write "工步号"(u32 30 ("变更工步号")) -> ()
                  }
                }
              }
              frame True {
                n242 = local write "工步号"(u32 40 ("变更工步号")) -> ()
              }
            }
          }
        }
      }
      frame 30 {
        # "人工调整"
        n243 = flat-sequence {
          tunnel: [w357] -> w355
          tunnel: w355 -> [w364]
          frame #0 {
            n244 = local write "测头机构轴速度(mm/s)"(30.0 ("测头机构轴速度(mm/s)")) -> ()
          }
          frame #1 {
            n245 = local read "测头机构电机"() -> (w358:u32)
            n246 = while {
              tunnel: w358 -> [w361]
              tunnel: [w360] -> w357
              stop <- w363 stop-if-true
              n247 = local read "测头机构轴待检位"() -> (w359:dbl)
              n248 = call "PCI1220U进给轴位置模式.vi"("Distance"=w359, "AxisHandle IN"=w361) -> ("AbsSuccess"=w363:bool, "AxisHandle OUT"=w360:u32)  [unwired: 8 in]
              n249 = Wait Until Next ms Multiple(millisecond multiple=u32 50 ("毫秒倍数")) -> ()  [unwired: 1 out]
            }
          }
          frame #2 {
            n250 = while {
              tunnel: w364 -> [w368]
              stop <- w366 stop-if-true
              n251 = call <userlib>:"Acm_AxGetCmdVelocity.vi"("AxisHandle"=w368) -> ("Velocity"=w367:dbl)  [unwired: 1 in, 3 out]
              n252 = Wait Until Next ms Multiple(millisecond multiple=u32 50 ("毫秒倍数")) -> ()  [unwired: 1 out]
              n253 = Equal To 0?(x=w367) -> (x = 0?=w366:bool)
            }
          }
          frame #3 {
            n254 = while {
              stop <- w370 stop-if-true
              n255 = local read "测头机构轴位置(mm)"() -> (w372:dbl)
              n256 = Wait Until Next ms Multiple(millisecond multiple=u32 50 ("毫秒倍数")) -> ()  [unwired: 1 out]
              n257 = Less Or Equal?(x=w372, y=35.0) -> (x <= y?=w370:bool)
            }
          }
          frame #4 {
            n258 = local write "测头气缸左移"(TRUE ("测头气缸左移")) -> ()
            n259 = local write "测头气缸右移"(FALSE ("测头气缸右移")) -> ()
          }
          frame #5 {
            n260 = while {
              stop <- w375 stop-if-true
              # "等待启动"
              n261 = local read "间隙启动"() -> (w375:bool)
              n262 = Wait Until Next ms Multiple(millisecond multiple=u32 50 ("毫秒倍数")) -> ()  [unwired: 1 out]
            }
          }
          frame #6 {
            n263 = local read "不合格品"() -> (w377:bool)
            n264 = case shown="真" w377 {
              frame False {
                n265 = flat-sequence {
                  frame #0 {
                    n266 = local read "单点间隙已调试次数"() -> (w380:dbl)
                    n267 = local write "测头气缸左移"(FALSE ("测头气缸左移")) -> ()
                    n268 = local write "测头气缸右移"(TRUE ("测头气缸左移")) -> ()
                    n269 = Add(x=w380, y=1.0 ("已调试次数")) -> (x+y=w382:dbl)
                    n270 = local write "单点间隙已调试次数"(w382) -> ()
                  }
                  frame #1 {
                    n271 = while {
                      stop <- w383 stop-if-true
                      n272 = Wait Until Next ms Multiple(millisecond multiple=u32 50 ("毫秒倍数")) -> ()  [unwired: 1 out]
                      n273 = local read "测头右位"() -> (w383:bool)
                    }
                  }
                  frame #2 {
                    n274 = local write "工步号"(u32 20 ("工步号")) -> ()
                  }
                }
              }
              frame True {
                n275 = local write "工步号"(u32 45 ("工步号")) -> ()
              }
            }
          }
        }
      }
      frame 40 {
        n276 = flat-sequence {
          tunnel: [w556] -> w552
          tunnel: w552 -> [w558]
          tunnel: [w557] -> w550
          tunnel: w550 -> [w564]
          tunnel: [w564] -> w394
          tunnel: w394 -> [w574]
          tunnel: [w574] -> w393
          tunnel: w393 -> [w576]
          tunnel: [w575] -> w392
          tunnel: w392 -> [w582]
          tunnel: [w582] -> w395
          tunnel: w395 -> [w591]
          tunnel: [w591] -> w541
          tunnel: w541 -> [w598]
          tunnel: [w598] -> w549
          tunnel: w549 -> [w600]
          tunnel: [w601] -> w482
          tunnel: [w599] -> w481
          tunnel: w482 -> [w612]
          tunnel: [w612] -> w478
          tunnel: w481 -> [w611]
          tunnel: [w611] -> w477
          tunnel: [w609] -> w469
          tunnel: [w608] -> w465
          tunnel: [w607] -> w461
          tunnel: w478 -> [w649]
          tunnel: [w649] -> w476
          tunnel: w477 -> [w648]
          tunnel: [w648] -> w474
          tunnel: [w647] -> w470
          tunnel: w469 -> [w647]
          tunnel: [w646] -> w466
          tunnel: w465 -> [w646]
          tunnel: [w645] -> w462
          tunnel: w461 -> [w645]
          tunnel: w476 -> [w655]
          tunnel: [w655] -> w475
          tunnel: w474 -> [w654]
          tunnel: [w654] -> w473
          tunnel: [w652] -> w471
          tunnel: w470 -> [w652]
          tunnel: [w651] -> w467
          tunnel: w466 -> [w651]
          tunnel: [w650] -> w463
          tunnel: w462 -> [w650]
          tunnel: w475 -> [w661]
          tunnel: [w661] -> w480
          tunnel: w473 -> [w660]
          tunnel: [w656] -> w479
          tunnel: [w659] -> w472
          tunnel: w471 -> [w659]
          tunnel: [w658] -> w468
          tunnel: w467 -> [w658]
          tunnel: [w657] -> w464
          tunnel: w463 -> [w657]
          tunnel: [w675] -> w546
          tunnel: [w674] -> w545
          tunnel: [w673] -> w544
          tunnel: w480 -> [w672]
          tunnel: [w672] -> w543
          tunnel: [w671] -> w542
          tunnel: w479 -> [w670]
          tunnel: w472 -> [w669]
          tunnel: w468 -> [w668]
          tunnel: w464 -> [w667]
          tunnel: w546 -> [w717]
          tunnel: [w717] -> w417
          tunnel: w545 -> [w724]
          tunnel: [w724] -> w415
          tunnel: w544 -> [w720]
          tunnel: [w720] -> w413
          tunnel: w543 -> [w723]
          tunnel: [w723] -> w411
          tunnel: [w719] -> w409
          tunnel: w542 -> [w719]
          tunnel: [w721] -> w407
          tunnel: [w709] -> w405
          tunnel: [w718] -> w403
          tunnel: [w710] -> w401
          tunnel: [w716] -> w399
          tunnel: w417 -> [w739]
          tunnel: [w739] -> w416
          tunnel: w415 -> [w738]
          tunnel: [w738] -> w414
          tunnel: w413 -> [w737]
          tunnel: [w737] -> w412
          tunnel: w411 -> [w736]
          tunnel: [w736] -> w410
          tunnel: w409 -> [w735]
          tunnel: [w735] -> w408
          tunnel: w407 -> [w734]
          tunnel: [w734] -> w406
          tunnel: w405 -> [w733]
          tunnel: [w733] -> w404
          tunnel: w403 -> [w732]
          tunnel: [w732] -> w402
          tunnel: w401 -> [w731]
          tunnel: [w731] -> w400
          tunnel: w399 -> [w730]
          tunnel: [w730] -> w398
          tunnel: w416 -> [w757]
          tunnel: [w757] -> w460
          tunnel: w414 -> [w756]
          tunnel: [w756] -> w459
          tunnel: w412 -> [w755]
          tunnel: [w740] -> w458
          tunnel: w410 -> [w754]
          tunnel: [w754] -> w457
          tunnel: [w753] -> w456
          tunnel: w408 -> [w753]
          tunnel: [w752] -> w455
          tunnel: w406 -> [w752]
          tunnel: w404 -> [w748]
          tunnel: w402 -> [w751]
          tunnel: w400 -> [w749]
          tunnel: w398 -> [w750]
          tunnel: [w750] -> w454
          tunnel: [w747] -> w453
          tunnel: [w742] -> w452
          tunnel: [w741] -> w451
          tunnel: w460 -> [w767]
          tunnel: w459 -> [w766]
          tunnel: w458 -> [w770]
          tunnel: [w769] -> w450
          tunnel: w457 -> [w771]
          tunnel: [w771] -> w449
          tunnel: w456 -> [w768]
          tunnel: [w764] -> w448
          tunnel: w455 -> [w776]
          tunnel: [w776] -> w447
          tunnel: w454 -> [w775]
          tunnel: [w775] -> w446
          tunnel: w453 -> [w774]
          tunnel: [w774] -> w445
          tunnel: w452 -> [w773]
          tunnel: [w773] -> w444
          tunnel: w451 -> [w772]
          tunnel: [w772] -> w443
          tunnel: [w765] -> w397
          tunnel: [w763] -> w391
          tunnel: [w811] -> w434
          tunnel: w450 -> [w809]
          tunnel: w449 -> [w818]
          tunnel: [w818] -> w431
          tunnel: w448 -> [w817]
          tunnel: [w817] -> w429
          tunnel: w447 -> [w816]
          tunnel: [w816] -> w427
          tunnel: w446 -> [w815]
          tunnel: [w815] -> w425
          tunnel: w445 -> [w814]
          tunnel: [w814] -> w423
          tunnel: w444 -> [w813]
          tunnel: [w813] -> w421
          tunnel: w443 -> [w812]
          tunnel: [w812] -> w419
          tunnel: w397 -> [w811]
          tunnel: w391 -> [w810]
          tunnel: [w810] -> w388
          tunnel: [w809] -> w387
          tunnel: w434 -> [w832]
          tunnel: [w832] -> w433
          tunnel: [w831] -> w432
          tunnel: w431 -> [w830]
          tunnel: [w830] -> w430
          tunnel: w429 -> [w829]
          tunnel: [w829] -> w428
          tunnel: w427 -> [w828]
          tunnel: [w828] -> w426
          tunnel: w425 -> [w827]
          tunnel: [w827] -> w424
          tunnel: w423 -> [w826]
          tunnel: [w826] -> w422
          tunnel: w421 -> [w825]
          tunnel: [w825] -> w420
          tunnel: w419 -> [w824]
          tunnel: [w824] -> w418
          tunnel: [w822] -> w389
          tunnel: w388 -> [w822]
          tunnel: w387 -> [w831]
          tunnel: w433 -> [w842]
          tunnel: [w842] -> w442
          tunnel: w432 -> [w833]
          tunnel: w430 -> [w841]
          tunnel: [w841] -> w441
          tunnel: w428 -> [w840]
          tunnel: [w840] -> w440
          tunnel: w426 -> [w839]
          tunnel: [w839] -> w439
          tunnel: w424 -> [w838]
          tunnel: [w838] -> w438
          tunnel: w422 -> [w837]
          tunnel: [w837] -> w437
          tunnel: w420 -> [w836]
          tunnel: [w836] -> w436
          tunnel: w418 -> [w835]
          tunnel: [w835] -> w435
          tunnel: [w833] -> w396
          tunnel: [w834] -> w390
          tunnel: w389 -> [w834]
          tunnel: [w860] -> w540
          tunnel: [w859] -> w539
          tunnel: w442 -> [w847]
          tunnel: [w858] -> w537
          tunnel: w441 -> [w850]
          tunnel: [w850] -> w535
          tunnel: w440 -> [w851]
          tunnel: w439 -> [w856]
          tunnel: [w857] -> w533
          tunnel: [w856] -> w531
          tunnel: w438 -> [w855]
          tunnel: [w855] -> w524
          tunnel: w437 -> [w854]
          tunnel: [w854] -> w509
          tunnel: w436 -> [w852]
          tunnel: w435 -> [w853]
          tunnel: [w853] -> w502
          tunnel: [w852] -> w501
          tunnel: w396 -> [w849]
          tunnel: w390 -> [w848]
          tunnel: w540 -> [w898]
          tunnel: w539 -> [w906]
          tunnel: [w906] -> w538
          tunnel: w537 -> [w902]
          tunnel: [w902] -> w536
          tunnel: w535 -> [w905]
          tunnel: [w905] -> w534
          tunnel: w533 -> [w904]
          tunnel: [w904] -> w532
          tunnel: w531 -> [w903]
          tunnel: [w903] -> w530
          tunnel: w524 -> [w899]
          tunnel: [w899] -> w523
          tunnel: [w898] -> w522
          tunnel: [w897] -> w521
          tunnel: [w896] -> w520
          tunnel: [w895] -> w510
          tunnel: w509 -> [w895]
          tunnel: w502 -> [w893]
          tunnel: w501 -> [w894]
          tunnel: [w894] -> w500
          tunnel: [w893] -> w499
          tunnel: w538 -> [w934]
          tunnel: [w949] -> w551
          tunnel: w536 -> [w949]
          tunnel: [w948] -> w547
          tunnel: w534 -> [w948]
          tunnel: w532 -> [w947]
          tunnel: w530 -> [w946]
          tunnel: [w944] -> w529
          tunnel: w523 -> [w943]
          tunnel: w522 -> [w942]
          tunnel: w521 -> [w940]
          tunnel: w520 -> [w939]
          tunnel: [w937] -> w519
          tunnel: [w936] -> w518
          tunnel: [w935] -> w517
          tunnel: w510 -> [w930]
          tunnel: [w930] -> w507
          tunnel: [w929] -> w504
          tunnel: [w928] -> w503
          tunnel: w500 -> [w927]
          tunnel: w499 -> [w926]
          tunnel: [w927] -> w498
          tunnel: [w926] -> w497
          tunnel: [w925] -> w492
          tunnel: [w924] -> w490
          tunnel: [w921] -> w487
          tunnel: [w916] -> w485
          tunnel: [w911] -> w483
          tunnel: w551 -> [w977]
          tunnel: [w977] -> w516
          tunnel: w547 -> [_]
          tunnel: [w973] -> w514
          tunnel: w529 -> [w975]
          tunnel: [w972] -> w512
          tunnel: w519 -> [w971]
          tunnel: w518 -> [w970]
          tunnel: w517 -> [w969]
          tunnel: [w968] -> w508
          tunnel: w507 -> [w968]
          tunnel: [w967] -> w506
          tunnel: [w966] -> w505
          tunnel: w504 -> [w965]
          tunnel: w503 -> [w964]
          tunnel: w498 -> [w959]
          tunnel: w497 -> [w958]
          tunnel: [w959] -> w496
          tunnel: [w958] -> w495
          tunnel: [w957] -> w494
          tunnel: [w956] -> w493
          tunnel: w492 -> [w956]
          tunnel: [w955] -> w491
          tunnel: w490 -> [w955]
          tunnel: [w954] -> w489
          tunnel: [w953] -> w488
          tunnel: w487 -> [w952]
          tunnel: [w951] -> w486
          tunnel: w485 -> [w951]
          tunnel: [w950] -> w484
          tunnel: w483 -> [w950]
          tunnel: w516 -> [w995]
          tunnel: [w995] -> w515
          tunnel: w514 -> [w994]
          tunnel: [w994] -> w513
          tunnel: w512 -> [w993]
          tunnel: [w993] -> w511
          tunnel: w508 -> [w989]
          tunnel: w506 -> [w987]
          tunnel: w505 -> [w986]
          tunnel: w496 -> [w990]
          tunnel: w495 -> [w988]
          tunnel: w494 -> [w985]
          tunnel: w493 -> [w984]
          tunnel: w491 -> [w983]
          tunnel: w489 -> [w982]
          tunnel: w488 -> [w981]
          tunnel: w486 -> [w979]
          tunnel: w484 -> [w978]
          tunnel: w515 -> [w999]
          tunnel: [w998] -> w548
          tunnel: w513 -> [w997]
          tunnel: w511 -> [w996]
          tunnel: [w996] -> w526
          tunnel: w548 -> [w1006]
          tunnel: [w1006] -> w528
          tunnel: w526 -> [w1005]
          tunnel: [w1005] -> w525
          tunnel: w528 -> [w1013]
          tunnel: [w1012] -> w527
          tunnel: w525 -> [w1011]
          tunnel: w527 -> [w1019]
          frame #0 {
            n277 = local write "选项卡控件"(T1."轴向力测量" ("选项卡控件")) -> ()
          }
          frame #1 {
            n278 = local write "电动缸速度(mm/s)"(15.0 ("电动缸速度(mm/s)")) -> ()
            n279 = local write "单点间隙已调试次数"(0.0 ("单点间隙已调试次数")) -> ()
            n280 = local read "电动缸电机"() -> (w556:u32)
          }
          frame #2 {
            n281 = while {
              tunnel: w558 -> [w563]
              tunnel: [w562] -> w557
              stop <- w561 stop-if-true
              n282 = local read "齿条左极限"() -> (w559:dbl)
              n283 = Wait (ms)(milliseconds to wait=u32 50 ("毫秒倍数")) -> ()  [unwired: 1 out]
              n284 = call "PCI1240电动缸位置模式 .vi"("Distance"=w559, "AxisHandle IN"=w563) -> ("AbsSuccess"=w561:bool, "AxisHandle OUT"=w562:u32)  [unwired: 8 in]
            }
          }
          frame #3 {
            n285 = while {
              tunnel: w564 -> [w572]
              stop <- w565 stop-if-true
              n286 = local read "齿条推拉力(N)"() -> (w569:dbl)
              n287 = call <userlib>:"Acm_AxGetCmdVelocity.vi"("AxisHandle"=w572) -> ("Velocity"=w571:dbl)  [unwired: 1 in, 3 out]
              n288 = Wait Until Next ms Multiple(millisecond multiple=u32 50 ("毫秒倍数")) -> ()  [unwired: 1 out]
              n289 = Equal To 0?(x=w571) -> (x = 0?=w567:bool)
              n290 = Less Or Equal?(x=w569, y=-500.0) -> (x <= y?=w566:bool)
              n291 = Or ("或")(x=w567, y=w566) -> (x .or. y?=w565:bool)
            }
          }
          frame #4 {
            n292 = local write "电动缸速度(mm/s)"(1.0 ("电动缸速度(mm/s)")) -> ()
          }
          frame #5 {
            n293 = while {
              tunnel: w576 -> [w581]
              tunnel: [w578] -> w575
              stop <- w579 stop-if-true
              n294 = Wait (ms)(milliseconds to wait=u32 50 ("毫秒倍数")) -> ()  [unwired: 1 out]
              n295 = call "PCI1240电动缸位置模式 .vi"("Distance"=10000.0, "AxisHandle IN"=w581) -> ("AbsSuccess"=w579:bool, "AxisHandle OUT"=w578:u32)  [unwired: 8 in]
            }
          }
          frame #6 {
            n296 = while {
              tunnel: w582 -> [w589]
              stop <- w583 stop-if-true
              n297 = local read "齿条推拉力(N)"() -> (w588:dbl)
              n298 = call <userlib>:"Acm_AxGetCmdVelocity.vi"("AxisHandle"=w589) -> ("Velocity"=w586:dbl)  [unwired: 1 in, 3 out]
              n299 = Wait Until Next ms Multiple(millisecond multiple=u32 50 ("毫秒倍数")) -> ()  [unwired: 1 out]
              n300 = Less Or Equal?(x=w588, y=-500.0) -> (x <= y?=w584:bool)
              n301 = Equal To 0?(x=w586) -> (x = 0?=w585:bool)
              n302 = Or ("或")(x=w585, y=w584) -> (x .or. y?=w583:bool)
            }
          }
          frame #7 {
            n303 = while {
              tunnel: w591 -> [w595]
              tunnel: [w594] -> _
              stop <- w593 stop-if-true
              n304 = call "PCI1220U停止.vi"("AxisHandle IN"=w595) -> ("完成"=w593:bool, "AxisHandle OUT"=w594:u32)  [unwired: 9 in]
              n305 = Wait (ms)(milliseconds to wait=u32 50 ("毫秒倍数")) -> ()  [unwired: 1 out]
            }
          }
          frame #8 {
            n306 = Wait Until Next ms Multiple(millisecond multiple=u32 50 ("毫秒倍数")) -> ()  [unwired: 1 out]
            n307 = local write "电动缸速度(mm/s)"(15.0 ("电动缸速度(mm/s)")) -> ()
          }
          frame #9 {
            n308 = while {
              tunnel: w600 -> [w606]
              tunnel: [w603] -> w599
              stop <- w604 stop-if-true
              n309 = local read "齿条右极限"() -> (w602:dbl)
              n310 = Wait Until Next ms Multiple(millisecond multiple=u32 50 ("毫秒倍数")) -> ()  [unwired: 1 out]
              n311 = call "PCI1240电动缸位置模式 .vi"("Distance"=w602, "AxisHandle IN"=w606) -> ("AbsSuccess"=w604:bool, "AxisHandle OUT"=w603:u32)  [unwired: 8 in]
            }
            n312 = local read "转向器中心"() -> (w601:dbl)
          }
          frame #10 {
            w610 = dbl[] []
            n313 = while {
              shift-right: [w632] -> w608
              shift-left: w610 -> [w643]
              shift-right: [w641] -> w609
              shift-left: w610 -> [w642]
              tunnel: w611 -> [w637]
              tunnel: [w637] -> _
              tunnel: w612 -> [w635]
              shift-right: [w631] -> w607
              shift-left: w610 -> [w633]
              stop <- w625 stop-if-true
              n314 = local read "中间位置间隙"() -> (w622:dbl)
              n315 = local read "基准位移"() -> (w638:dbl)
              n316 = local read "间隙位移(mm)"() -> (w621:dbl)
              n317 = call <userlib>:"Acm_AxGetCmdVelocity.vi"("AxisHandle"=w637) -> ("Velocity"=w630:dbl)  [unwired: 1 in, 3 out]
              n318 = Wait (ms)(milliseconds to wait=u32 50 ("毫秒倍数")) -> ()  [unwired: 1 out]
              n319 = local read "齿条推拉力(N)"() -> (w628:dbl)
              n320 = call "PCI1240电动缸读取位置.vi"("AxisHandle IN"=w637) -> ("位置"=w636:dbl)  [unwired: 9 in, 1 out]
              n321 = Subtract(x=w621, y=w638) -> (x-y=w624:dbl)
              n322 = Subtract(x=w636, y=w635) -> (x-y=w615:dbl)
              n323 = Add(x=w624, y=w622) -> (x+y=w623:dbl)
              n324 = Multiply(x=w615, y=1.12) -> (x*y=w613:dbl)
              n325 = Build Array (concatenate) ("创建数组")(w642, w623) -> (w641:dbl[])
              n326 = Build Array (concatenate) ("创建数组")(w643, w613) -> (w632:dbl[])
              n327 = Build Array (concatenate) ("创建数组")(w633, w628) -> (w631:dbl[])
              n328 = Greater Or Equal?(x=w628, y=500.0) -> (x >= y?=w626:bool)
              n329 = Less Or Equal?(x=w621, y=-1.0) -> (x <= y?=w620:bool)
              n330 = Greater Or Equal?(x=w621, y=4.0) -> (x >= y?=w619:bool)
              n331 = Equal To 0?(x=w630) -> (x = 0?=w627:bool)
              n332 = Or(x=w619, y=w620) -> (x .or. y?=w618:bool)
              n333 = Bundle ("捆绑")(w632, w641) -> (w639:cluster{dbl[], dbl[]})  [unwired: 1 in]
              n334 = Or(x=w627, y=w626) -> (x .or. y?=w625:bool)
              n335 = Bundle ("捆绑")(w632, w631) -> (w634:cluster{dbl[], dbl[]})  [unwired: 1 in]
              n336 = property on="间隙位移(mm)" class="DigNum (严格)"("Blinking"=w618) -> ()  [unwired: 2 in, 2 out]
              n337 = Build Array ("创建数组")(w639, w634) -> (w640:cluster{dbl[], dbl[]}[])
              n338 = local write "行程跳动曲线"(w640) -> ()
            }
          }
          frame #11 {
            n339 = call "PCI1220U停止.vi"("AxisHandle IN"=w648) -> ()  [unwired: 9 in, 2 out]
          }
          frame #12 {
            n340 = local write "电动缸速度(mm/s)"(1.0 ("电动缸速度(mm/s)")) -> ()
          }
          frame #13 {
            n341 = while {
              tunnel: w660 -> [w666]
              tunnel: [w663] -> w656
              stop <- w664 stop-if-true
              # "该位置为最右边"
              n342 = Wait Until Next ms Multiple(millisecond multiple=u32 50 ("毫秒倍数")) -> ()  [unwired: 1 out]
              n343 = call "PCI1240电动缸位置模式 .vi"("Distance"=10.0, "AxisHandle IN"=w666) -> ("AbsSuccess"=w664:bool, "AxisHandle OUT"=w663:u32)  [unwired: 8 in]
            }
          }
          frame #14 {
            n344 = while {
              shift-right: [w695] -> w674
              shift-left: w668 -> [w706]
              shift-right: [w704] -> w675
              shift-left: w669 -> [w705]
              tunnel: w670 -> [w700]
              tunnel: [w700] -> w673
              tunnel: w672 -> [w698]
              shift-right: [w694] -> w671
              shift-left: w667 -> [w696]
              stop <- w688 stop-if-true
              n345 = local read "中间位置间隙"() -> (w685:dbl)
              n346 = local read "基准位移"() -> (w701:dbl)
              n347 = local read "间隙位移(mm)"() -> (w684:dbl)
              n348 = call <userlib>:"Acm_AxGetCmdVelocity.vi"("AxisHandle"=w700) -> ("Velocity"=w693:dbl)  [unwired: 1 in, 3 out]
              n349 = Wait (ms)(milliseconds to wait=u32 50 ("毫秒倍数")) -> ()  [unwired: 1 out]
              n350 = local read "齿条推拉力(N)"() -> (w691:dbl)
              n351 = call "PCI1240电动缸读取位置.vi"("AxisHandle IN"=w700) -> ("位置"=w699:dbl)  [unwired: 9 in, 1 out]
              n352 = Subtract(x=w684, y=w701) -> (x-y=w687:dbl)
              n353 = Subtract(x=w699, y=w698) -> (x-y=w678:dbl)
              n354 = Add(x=w687, y=w685) -> (x+y=w686:dbl)
              n355 = Multiply(x=w678, y=1.12) -> (x*y=w676:dbl)
              n356 = Build Array (concatenate) ("创建数组")(w705, w686) -> (w704:dbl[])
              n357 = Build Array (concatenate) ("创建数组")(w706, w676) -> (w695:dbl[])
              n358 = Build Array (concatenate) ("创建数组")(w696, w691) -> (w694:dbl[])
              n359 = Greater Or Equal?(x=w691, y=500.0) -> (x >= y?=w689:bool)
              n360 = Less Or Equal?(x=w684, y=-1.0) -> (x <= y?=w683:bool)
              n361 = Greater Or Equal?(x=w684, y=4.0) -> (x >= y?=w682:bool)
              n362 = Equal To 0?(x=w693) -> (x = 0?=w690:bool)
              n363 = Or(x=w682, y=w683) -> (x .or. y?=w681:bool)
              n364 = Bundle ("捆绑")(w695, w704) -> (w702:cluster{dbl[], dbl[]})  [unwired: 1 in]
              n365 = Or(x=w690, y=w689) -> (x .or. y?=w688:bool)
              n366 = Bundle ("捆绑")(w695, w694) -> (w697:cluster{dbl[], dbl[]})  [unwired: 1 in]
              n367 = property on="间隙位移(mm)" class="DigNum (严格)"("Blinking"=w681) -> ()  [unwired: 2 in, 2 out]
              n368 = Build Array ("创建数组")(w702, w697) -> (w703:cluster{dbl[], dbl[]}[])
              n369 = local write "行程跳动曲线"(w703) -> ()
            }
          }
          frame #15 {
            n370 = while {
              tunnel: w720 -> [w728]
              tunnel: [w727] -> _
              stop <- w726 stop-if-true
              n371 = call "PCI1220U停止.vi"("AxisHandle IN"=w728) -> ("完成"=w726:bool, "AxisHandle OUT"=w727:u32)  [unwired: 9 in]
              n372 = Wait (ms)(milliseconds to wait=u32 50 ("毫秒倍数")) -> ()  [unwired: 1 out]
            }
            n373 = Array Size(array=w719) -> (size(s)=w721:i32)
            n374 = Array Size(array=w717) -> (size(s)=w716:i32)
            n375 = Wait Until Next ms Multiple(millisecond multiple=u32 500 ("毫秒倍数")) -> ()  [unwired: 1 out]
            n376 = call "功能计算.vi"("扭矩数组"=w719) -> ("扭差"=w710:dbl, "平均扭矩"=w718:dbl, "峰值扭矩"=w709:dbl)  [unwired: 7 in, 1 out]
            "左轴向力波动(N)" <- w710
            "左最大轴向力(N)" <- w709
            n377 = call "间隙计算.vi"("扭矩数组"=w717) -> ("峰值间隙1"=w715:dbl, "峰值间隙2"=w714:dbl)  [unwired: 6 in, 3 out]
            n378 = local read "180°内全行程间隙标准(mm)"() -> (w713:dbl)
            n379 = local read "180°外全行程间隙标准(mm)"() -> (w708:dbl)
            n380 = local write "左平均轴向力(N)"(w718) -> ()
            n381 = local write "左180°外全行程间隙"(w714) -> ()
            n382 = local write "左180°内全行程间隙"(w715) -> ()
            n383 = Greater?(x=w715, y=w713) -> (0:w712:bool)
            n384 = Greater?(x=w714, y=w708) -> (0:w711:bool)
            n385 = property on="左180°内全行程间隙" class="DigNum (严格)"("Blinking"=w712) -> ()  [unwired: 2 in, 2 out]
            n386 = property on="左180°外全行程间隙" class="DigNum (严格)"("Blinking"=w711) -> ()  [unwired: 2 in, 2 out]
          }
          frame #16 {
            n387 = local write "电动缸速度(mm/s)"(15.0 ("电动缸速度(mm/s)")) -> ()
          }
          frame #17 {
            n388 = local read "最大轴向力标准(N)"() -> (w746:dbl)
            n389 = local read "平均轴向力标准(N)"() -> (w745:dbl)
            n390 = while {
              tunnel: w755 -> [w762]
              tunnel: w754 -> [_]
              tunnel: [w758] -> w740
              stop <- w761 stop-if-true
              n391 = Wait Until Next ms Multiple(millisecond multiple=u32 50 ("毫秒倍数")) -> ()  [unwired: 1 out]
              n392 = local read "齿条左极限"() -> (w759:dbl)
              n393 = call "PCI1240电动缸位置模式 .vi"("Distance"=w759, "AxisHandle IN"=w762) -> ("AbsSuccess"=w761:bool, "AxisHandle OUT"=w758:u32)  [unwired: 8 in]
            }
            n394 = local read "平均轴向力标准(N) max"() -> (w744:dbl)
            n395 = local read "力波动标准(N)"() -> (w743:dbl)
            n396 = call "判断.vi"("y 3"=w743, "y 2-2"=w744, "y 2-1"=w745, "y"=w746, "x 3"=w749, "x 2"=w751, "x"=w748) -> ("非x? 3"=w741:bool, "非x? 2"=w747:bool, "非x?"=w742:bool)  [unwired: 2 in]
            n397 = property on="左最大轴向力(N)" class="DigNum (严格)"("Blinking"=w742) -> ()  [unwired: 2 in, 2 out]
            n398 = property on="左平均轴向力(N)" class="DigNum (严格)"("Blinking"=w747) -> ()  [unwired: 2 in, 2 out]
            n399 = property on="左轴向力波动(N)" class="DigNum (严格)"("Blinking"=w741) -> ()  [unwired: 2 in, 2 out]
          }
          frame #18 {
            n400 = while {
              shift-right: [w797] -> w763
              shift-left: w766 -> [w807]
              shift-right: [w805] -> w765
              shift-left: w767 -> [w806]
              tunnel: w770 -> [w800]
              tunnel: [w800] -> w769
              tunnel: w771 -> [w798]
              shift-right: [w794] -> w764
              shift-left: w768 -> [w795]
              stop <- w789 stop-if-true
              n401 = call <userlib>:"Acm_AxGetCmdVelocity.vi"("AxisHandle"=w800) -> ("Velocity"=w787:dbl)  [unwired: 1 in, 3 out]
              n402 = local read "间隙位移(mm)"() -> (w781:dbl)
              n403 = local read "基准位移"() -> (w801:dbl)
              n404 = Wait (ms)(milliseconds to wait=u32 50 ("毫秒倍数")) -> ()  [unwired: 1 out]
              n405 = local read "中间位置间隙"() -> (w786:dbl)
              n406 = local read "齿条推拉力(N)"() -> (w793:dbl)
              n407 = call "PCI1240电动缸读取位置.vi"("AxisHandle IN"=w800) -> ("位置"=w799:dbl)  [unwired: 9 in, 1 out]
              n408 = Subtract(x=w781, y=w801) -> (x-y=w802:dbl)
              n409 = Subtract(x=w799, y=w798) -> (x-y=w779:dbl)
              n410 = Add(x=w802, y=w786) -> (x+y=w788:dbl)
              n411 = Multiply(x=w779, y=1.12) -> (x*y=w777:dbl)
              n412 = Build Array (concatenate) ("创建数组")(w807, w777) -> (w797:dbl[])
              n413 = Less Or Equal?(x=w793, y=-500.0) -> (x <= y?=w790:bool)
              n414 = Build Array (concatenate) ("创建数组")(w795, w793) -> (w794:dbl[])
              n415 = Equal To 0?(x=w787) -> (x = 0?=w791:bool)
              n416 = Build Array (concatenate) ("创建数组")(w806, w788) -> (w805:dbl[])
              n417 = Bundle ("捆绑")(w797, w794) -> (w796:cluster{dbl[], dbl[]})  [unwired: 1 in]
              n418 = Or(x=w791, y=w790) -> (x .or. y?=w789:bool)
              n419 = Bundle ("捆绑")(w797, w805) -> (w803:cluster{dbl[], dbl[]})  [unwired: 1 in]
              n420 = Build Array ("创建数组")(w803, w796) -> (w804:cluster{dbl[], dbl[]}[])
              n421 = Less Or Equal?(x=w781, y=-1.0) -> (x <= y?=w785:bool)
              n422 = Greater Or Equal?(x=w781, y=4.0) -> (x >= y?=w784:bool)
              n423 = local write "行程跳动曲线"(w804) -> ()
              n424 = Or(x=w784, y=w785) -> (x .or. y?=w780:bool)
              n425 = property on="间隙位移(mm)" class="DigNum (严格)"("Blinking"=w780) -> ()  [unwired: 2 in, 2 out]
            }
          }
          frame #19 {
            n426 = while {
              tunnel: w809 -> [w821]
              stop <- w820 stop-if-true
              n427 = call "PCI1220U停止.vi"("AxisHandle IN"=w821) -> ("完成"=w820:bool)  [unwired: 9 in, 1 out]
              n428 = Wait (ms)(milliseconds to wait=u32 50 ("毫秒倍数")) -> ()  [unwired: 1 out]
            }
          }
          frame #20 {
            n429 = local write "电动缸速度(mm/s)"(1.0 ("电动缸速度(mm/s)")) -> ()
          }
          frame #21 {
            n430 = while {
              tunnel: w833 -> [w846]
              stop <- w844 stop-if-true
              # "该位置为最左边"
              n431 = Wait Until Next ms Multiple(millisecond multiple=u32 50 ("毫秒倍数")) -> ()  [unwired: 1 out]
              n432 = call "PCI1240电动缸位置模式 .vi"("Distance"=160.0, "AxisHandle IN"=w846) -> ("AbsSuccess"=w844:bool)  [unwired: 8 in, 1 out]
            }
          }
          frame #22 {
            n433 = while {
              shift-right: [w881] -> w859
              shift-left: w848 -> [w891]
              shift-right: [w889] -> w860
              shift-left: w847 -> [w890]
              tunnel: w849 -> [w884]
              tunnel: [w884] -> w858
              tunnel: w850 -> [w882]
              shift-right: [w878] -> w857
              shift-left: w851 -> [w879]
              stop <- w873 stop-if-true
              n434 = call <userlib>:"Acm_AxGetCmdVelocity.vi"("AxisHandle"=w884) -> ("Velocity"=w871:dbl)  [unwired: 1 in, 3 out]
              n435 = local read "间隙位移(mm)"() -> (w865:dbl)
              n436 = local read "基准位移"() -> (w885:dbl)
              n437 = Wait (ms)(milliseconds to wait=u32 50 ("毫秒倍数")) -> ()  [unwired: 1 out]
              n438 = local read "中间位置间隙"() -> (w870:dbl)
              n439 = local read "齿条推拉力(N)"() -> (w877:dbl)
              n440 = call "PCI1240电动缸读取位置.vi"("AxisHandle IN"=w884) -> ("位置"=w883:dbl)  [unwired: 9 in, 1 out]
              n441 = Subtract(x=w865, y=w885) -> (x-y=w886:dbl)
              n442 = Subtract(x=w883, y=w882) -> (x-y=w863:dbl)
              n443 = Add(x=w886, y=w870) -> (x+y=w872:dbl)
              n444 = Multiply(x=w863, y=1.12) -> (x*y=w861:dbl)
              n445 = Build Array (concatenate) ("创建数组")(w891, w861) -> (w881:dbl[])
              n446 = Less Or Equal?(x=w877, y=-500.0) -> (x <= y?=w874:bool)
              n447 = Build Array (concatenate) ("创建数组")(w879, w877) -> (w878:dbl[])
              n448 = Equal To 0?(x=w871) -> (x = 0?=w875:bool)
              n449 = Build Array (concatenate) ("创建数组")(w890, w872) -> (w889:dbl[])
              n450 = Bundle ("捆绑")(w881, w878) -> (w880:cluster{dbl[], dbl[]})  [unwired: 1 in]
              n451 = Or(x=w875, y=w874) -> (x .or. y?=w873:bool)
              n452 = Bundle ("捆绑")(w881, w889) -> (w887:cluster{dbl[], dbl[]})  [unwired: 1 in]
              n453 = Build Array ("创建数组")(w887, w880) -> (w888:cluster{dbl[], dbl[]}[])
              n454 = Less Or Equal?(x=w865, y=-1.0) -> (x <= y?=w869:bool)
              n455 = Greater Or Equal?(x=w865, y=4.0) -> (x >= y?=w868:bool)
              n456 = local write "行程跳动曲线"(w888) -> ()
              n457 = Or(x=w868, y=w869) -> (x .or. y?=w864:bool)
              n458 = property on="间隙位移(mm)" class="DigNum (严格)"("Blinking"=w864) -> ()  [unwired: 2 in, 2 out]
            }
          }
          frame #23 {
            n459 = while {
              tunnel: w902 -> [w910]
              tunnel: [w909] -> _
              stop <- w908 stop-if-true
              n460 = call "PCI1220U停止.vi"("AxisHandle IN"=w910) -> ("完成"=w908:bool, "AxisHandle OUT"=w909:u32)  [unwired: 9 in]
              n461 = Wait (ms)(milliseconds to wait=u32 50 ("毫秒倍数")) -> ()  [unwired: 1 out]
            }
            n462 = Array Max & Min(array=w898) -> (max value=w901:dbl, min value=w900:dbl)  [unwired: 2 out]
            n463 = Absolute Value(x=w901) -> (abs(x)=w897:dbl)
            n464 = Absolute Value(x=w900) -> (abs(x)=w896:dbl)
            n465 = local write "左全行程间隙"(w897) -> ()
            n466 = local write "右全行程间隙"(w896) -> ()
          }
          frame #24 {
            n467 = local read "180°内全行程间隙标准(mm)"() -> (w938:dbl)
            n468 = Split 1D Array(array=w947, index=w946) -> (second subarray=w945:dbl[])  [unwired: 1 out]
            n469 = Array Max & Min(array=w934) -> (max value=w933:dbl, min value=w932:dbl)  [unwired: 2 out]
            n470 = local read "机械间隙值"() -> (w922:dbl)
            n471 = local read "总圈数标准"() -> (w914:dbl)
            n472 = local read "总圈数最大值"() -> (w915:dbl)
            n473 = Subtract(x=w933, y=w932) -> (x-y=w923:dbl)
            n474 = call "功能计算.vi"("扭矩数组"=w945) -> ("扭差"=w928:dbl, "平均扭矩"=w944:dbl, "峰值扭矩"=w929:dbl)  [unwired: 7 in, 1 out]
            n475 = Subtract(x=w923, y=w922) -> (x-y=w920:dbl)
            n476 = Split 1D Array(array=w942, index=w943) -> (second subarray=w941:dbl[])  [unwired: 1 out]
            n477 = Greater?(x=w940, y=w938) -> (0:w925:bool)
            n478 = Greater?(x=w939, y=w938) -> (0:w924:bool)
            n479 = local write "右最大轴向力(N)"(w929) -> ()
            n480 = call "间隙计算.vi"("扭矩数组"=w941) -> ("峰值间隙1"=w936:dbl, "峰值间隙2"=w935:dbl)  [unwired: 6 in, 3 out]
            n481 = Divide(x=w920, y=46.996) -> (x/y=w913:dbl)
            n482 = In Range and Coerce(upper limit=w915, x=w913, lower limit=w914) -> (In Range?=w912:bool)  [unwired: 1 out]
            n483 = Not(x=w912) -> (.not. x?=w911:bool)
            n484 = property on="总圈数" class="DigNum (严格)"("Blinking"=w911) -> ()  [unwired: 2 in, 2 out]
            n485 = property on="左全行程间隙" class="DigNum (严格)"("Blinking"=w925) -> ()  [unwired: 2 in, 2 out]
            n486 = property on="右全行程间隙" class="DigNum (严格)"("Blinking"=w924) -> ()  [unwired: 2 in, 2 out]
            n487 = local write "右平均轴向力(N)"(w944) -> ()
            n488 = local write "右轴向力波动(N)"(w928) -> ()
            n489 = local write "总圈数"(w913) -> ()
            n490 = local read "180°内全行程间隙标准(mm)"() -> (w937:dbl)
            n491 = local read "总行程标准(mm)"() -> (w918:dbl)
            n492 = local read "总行程最大值"() -> (w919:dbl)
            n493 = In Range and Coerce(upper limit=w919, x=w920, lower limit=w918) -> (In Range?=w917:bool)  [unwired: 1 out]
            n494 = local write "右180°外全行程间隙"(w935) -> ()
            n495 = local write "右180°内全行程间隙"(w936) -> ()
            n496 = local read "180°外全行程间隙标准(mm)"() -> (w921:dbl)
            n497 = Not(x=w917) -> (.not. x?=w916:bool)
            n498 = local write "总行程"(w920) -> ()
            n499 = property on="总行程" class="DigNum (严格)"("Blinking"=w916) -> ()  [unwired: 2 in, 2 out]
            "轴向力X" <- w934
            "轴向力Y" <- w947
          }
          frame #25 {
            n500 = local read "最大轴向力标准(N)"() -> (w963:dbl)
            n501 = local read "平均轴向力标准(N)"() -> (w962:dbl)
            n502 = local read "平均轴向力标准(N) max"() -> (w961:dbl)
            n503 = Greater?(x=w970, y=w971) -> (0:w954:bool)
            n504 = Greater?(x=w969, y=w952) -> (0:w953:bool)
            n505 = local write "电动缸速度(mm/s)"(15.0 ("电动缸速度(mm/s)")) -> ()
            n506 = local read "转向器中心"() -> (w972:dbl)
            n507 = local read "力波动标准(N)"() -> (w960:dbl)
            n508 = call "判断.vi"("y 3"=w960, "y 2-2"=w961, "y 2-1"=w962, "y"=w963, "x 3"=w964, "x 2"=w975, "x"=w965) -> ("非x? 3"=w957:bool, "非x? 2"=w966:bool, "非x?"=w967:bool)  [unwired: 2 in]
            n509 = property on="右180°内全行程间隙" class="DigNum (严格)"("Blinking"=w954) -> ()  [unwired: 2 in, 2 out]
            n510 = property on="右180°外全行程间隙" class="DigNum (严格)"("Blinking"=w953) -> ()  [unwired: 2 in, 2 out]
            n511 = Add(x=w972, y=-10.0) -> (x+y=w973:dbl)
          }
          frame #26 {
            n512 = Compound Arithmetic op=OR(w984, w983, w982, w981) -> (w980:bool)
            n513 = property on="右最大轴向力(N)" class="DigNum (严格)"("Blinking"=w987) -> ()  [unwired: 2 in, 2 out]
            n514 = property on="右平均轴向力(N)" class="DigNum (严格)"("Blinking"=w986) -> ()  [unwired: 2 in, 2 out]
            n515 = property on="右轴向力波动(N)" class="DigNum (严格)"("Blinking"=w985) -> ()  [unwired: 2 in, 2 out]
            n516 = Compound Arithmetic op=OR(w978, w980, w987, w986, w985, w990, w989, w988, w979) -> (w992:bool)
            n517 = Not(x=w992) -> (.not. x?=w991:bool)
            n518 = local write "轴向力及全行程间隙合格"(w991) -> ()
          }
          frame #27 {
            n519 = while {
              tunnel: w999 -> [w1003]
              tunnel: [w1001] -> w998
              tunnel: w997 -> [w1000]
              stop <- w1002 stop-if-true
              n520 = call "PCI1240电动缸位置模式 .vi"("Distance"=w1000, "AxisHandle IN"=w1003) -> ("AbsSuccess"=w1002:bool, "AxisHandle OUT"=w1001:u32)  [unwired: 8 in]
              n521 = Wait (ms)(milliseconds to wait=u32 50 ("毫秒倍数")) -> ()  [unwired: 1 out]
            }
          }
          frame #28 {
            n522 = while {
              tunnel: w1006 -> [w1010]
              stop <- w1008 stop-if-true
              n523 = call <userlib>:"Acm_AxGetCmdVelocity.vi"("AxisHandle"=w1010) -> ("Velocity"=w1009:dbl)  [unwired: 1 in, 3 out]
              n524 = Wait Until Next ms Multiple(millisecond multiple=u32 50 ("毫秒倍数")) -> ()  [unwired: 1 out]
              n525 = Equal To 0?(x=w1009) -> (x = 0?=w1008:bool)
            }
          }
          frame #29 {
            n526 = while {
              tunnel: w1013 -> [w1017]
              tunnel: [w1015] -> w1012
              tunnel: w1011 -> [w1014]
              stop <- w1016 stop-if-true
              n527 = call "PCI1240电动缸位置模式 .vi"("Distance"=w1014, "AxisHandle IN"=w1017) -> ("AbsSuccess"=w1016:bool, "AxisHandle OUT"=w1015:u32)  [unwired: 8 in]
              n528 = Wait (ms)(milliseconds to wait=u32 50 ("毫秒倍数")) -> ()  [unwired: 1 out]
            }
          }
          frame #30 {
            n529 = while {
              tunnel: w1019 -> [w1023]
              stop <- w1021 stop-if-true
              n530 = call <userlib>:"Acm_AxGetCmdVelocity.vi"("AxisHandle"=w1023) -> ("Velocity"=w1022:dbl)  [unwired: 1 in, 3 out]
              n531 = Wait Until Next ms Multiple(millisecond multiple=u32 50 ("毫秒倍数")) -> ()  [unwired: 1 out]
              n532 = Equal To 0?(x=w1022) -> (x = 0?=w1021:bool)
            }
          }
          frame #31 {
            n533 = local read "轴向力已做次数"() -> (w1026:dbl)
            n534 = Add(x=w1026, y=1.0) -> (x+y=w1024:dbl)
            n535 = local write "轴向力已做次数"(w1024) -> ()
          }
          frame #32 {
            n536 = local read "轴向力及全行程间隙合格"() -> (w1027:bool)
            n537 = case shown="假" w1027 {
              frame False {
                n538 = Less?(x="轴向力已做次数", y="轴向力设定次数") -> (x < y?=w1029:bool)
                n539 = case shown="真" w1029 {
                  frame False {
                    n540 = local write "工步号"(u32 45 ("工步号")) -> ()
                  }
                  frame True {
                    n541 = local write "工步号"(u32 30 ("工步号")) -> ()
                  }
                }
              }
              frame True {
                n542 = local write "工步号"(u32 45 ("工步号")) -> ()
              }
            }
          }
        }
      }
      frame 45 {
        # "测头退回"
        n543 = flat-sequence {
          tunnel: [w1037] -> w1034
          tunnel: w1034 -> [w1044]
          frame #0 {
            n544 = local write "测头机构轴速度(mm/s)"(30.0 ("测头机构轴速度(mm/s)")) -> ()
          }
          frame #1 {
            n545 = local read "测头机构轴后退位"() -> (w1036:dbl)
            n546 = local read "测头机构电机"() -> (w1038:u32)
            n547 = while {
              tunnel: w1038 -> [w1042]
              tunnel: w1036 -> [w1041]
              tunnel: [w1040] -> w1037
              stop <- w1043 stop-if-true
              n548 = Wait Until Next ms Multiple(millisecond multiple=u32 50 ("毫秒倍数")) -> ()  [unwired: 1 out]
              n549 = call "PCI1220U进给轴位置模式.vi"("Distance"=w1041, "AxisHandle IN"=w1042) -> ("AbsSuccess"=w1043:bool, "AxisHandle OUT"=w1040:u32)  [unwired: 8 in]
            }
          }
          frame #2 {
            n550 = while {
              tunnel: w1044 -> [w1048]
              stop <- w1046 stop-if-true
              n551 = call <userlib>:"Acm_AxGetCmdVelocity.vi"("AxisHandle"=w1048) -> ("Velocity"=w1047:dbl)  [unwired: 1 in, 3 out]
              n552 = Wait Until Next ms Multiple(millisecond multiple=u32 50 ("毫秒倍数")) -> ()  [unwired: 1 out]
              n553 = Equal To 0?(x=w1047) -> (x = 0?=w1046:bool)
            }
          }
          frame #3 {
            n554 = while {
              stop <- w1050 stop-if-true
              n555 = local read "测头机构轴位置(mm)"() -> (w1052:dbl)
              n556 = Wait Until Next ms Multiple(millisecond multiple=u32 50 ("毫秒倍数")) -> ()  [unwired: 1 out]
              n557 = Less Or Equal?(x=w1052, y=35.0) -> (x <= y?=w1050:bool)
            }
          }
          frame #4 {
            n558 = local write "测头气缸右移"(FALSE ("测头气缸右移")) -> ()
            n559 = local write "测头气缸左移"(TRUE ("测头气缸左移")) -> ()
          }
          frame #5 {
            n560 = Wait Until Next ms Multiple(millisecond multiple=u32 500 ("毫秒倍数")) -> ()  [unwired: 1 out]
          }
          frame #6 {
            n561 = local write "工步号"(u32 50 ("工步号")) -> ()
          }
        }
      }
      frame 50 {
        n562 = flat-sequence {
          tunnel: [w1079] -> w1068
          tunnel: w1068 -> [w1086]
          tunnel: [w1085] -> w1065
          tunnel: w1065 -> [w1097]
          tunnel: [w1103] -> w1062
          tunnel: w1062 -> [w1106]
          tunnel: [w1105] -> w1061
          tunnel: w1061 -> [w1110]
          tunnel: [w1110] -> w1060
          tunnel: w1060 -> [w1112]
          tunnel: [w1111] -> w1058
          tunnel: [w1118] -> w1059
          tunnel: w1058 -> [w1119]
          tunnel: w1059 -> [w1121]
          tunnel: [w1120] -> w1057
          tunnel: [w1127] -> w1067
          tunnel: w1057 -> [w1127]
          tunnel: w1067 -> [w1130]
          tunnel: [w1129] -> w1066
          tunnel: w1066 -> [w1136]
          tunnel: [w1137] -> w1064
          tunnel: w1064 -> [w1144]
          tunnel: [w1143] -> w1063
          tunnel: w1063 -> [w1154]
          frame #0 {
            n563 = local write "旋转齿条轴速度(°/s)"(15.0 ("调整螺塞轴速度(°/s)")) -> ()
            n564 = local write "测头机构轴速度(mm/s)"(15.0 ("调整机构轴速度(mm/s)")) -> ()
            n565 = local write "电动缸速度(mm/s)"(15.0 ("电动缸速度(mm/s)")) -> ()
            n566 = local write "夹头夹紧"(FALSE ("夹头夹紧")) -> ()
            n567 = local write "夹头松开"(TRUE ("夹头松开")) -> ()
          }
          frame #1 {
            n568 = while {
              stop <- w1074 stop-if-true
              n569 = local read "夹头松开"() -> (w1075:bool)
              n570 = local read "夹头夹紧"() -> (w1077:bool)
              n571 = Wait Until Next ms Multiple(millisecond multiple=u32 50 ("毫秒倍数")) -> ()  [unwired: 1 out]
              n572 = Not(x=w1077) -> (.not. x?=w1076:bool)
              n573 = And(x=w1076, y=w1075) -> (x .and. y?=w1074:bool)
            }
          }
          frame #2 {
            n574 = while {
              tunnel: [w1082] -> w1079
              stop <- w1081 stop-if-true
              n575 = local read "电动缸电机"() -> (w1083:u32)
              n576 = Wait Until Next ms Multiple(millisecond multiple=u32 50 ("毫秒倍数")) -> ()  [unwired: 1 out]
              n577 = local read "齿条右极限"() -> (w1080:dbl)
              n578 = call "PCI1240电动缸位置模式 .vi"("Distance"=w1080, "AxisHandle IN"=w1083) -> ("AbsSuccess"=w1081:bool, "AxisHandle OUT"=w1082:u32)  [unwired: 8 in]
            }
          }
          frame #3 {
            n579 = while {
              tunnel: w1086 -> [w1095]
              tunnel: [w1087] -> w1085
              stop <- w1088 stop-if-true
              n580 = local read "齿条推拉力(N)"() -> (w1093:dbl)
              n581 = Wait Until Next ms Multiple(millisecond multiple=u32 50 ("毫秒倍数")) -> ()  [unwired: 1 out]
              n582 = call <userlib>:"Acm_AxGetCmdVelocity.vi"("AxisHandle"=w1095) -> ("Velocity"=w1096:dbl, "AxisHandle"=w1087:u32)  [unwired: 1 in, 2 out]
              n583 = Equal To 0?(x=w1096) -> (x = 0?=w1090:bool)
              n584 = Absolute Value(x=w1093) -> (abs(x)=w1092:dbl)
              n585 = Greater Or Equal?(x=w1092, y=1000.0) -> (x >= y?=w1089:bool)
              n586 = Or(x=w1090, y=w1089) -> (x .or. y?=w1088:bool)
            }
          }
          frame #4 {
            n587 = while {
              tunnel: w1097 -> [w1101]
              tunnel: [w1100] -> _
              stop <- w1099 stop-if-true
              n588 = call "PCI1220U停止.vi"("AxisHandle IN"=w1101) -> ("完成"=w1099:bool, "AxisHandle OUT"=w1100:u32)  [unwired: 9 in]
              n589 = Wait (ms)(milliseconds to wait=u32 50 ("毫秒倍数")) -> ()  [unwired: 1 out]
            }
          }
          frame #5 {
            n590 = local write "旋转齿条轴使能"(TRUE ("旋转齿条轴使能")) -> ()
          }
          frame #6 {
            n591 = local read "旋转齿条电机"() -> (w1103:u32)
            n592 = Wait Until Next ms Multiple(millisecond multiple=u32 500 ("毫秒倍数")) -> ()  [unwired: 1 out]
          }
          frame #7 {
            n593 = call <userlib>:"Acm_AxHome.vi"("DirMode"=u32 0, "HomeMode"=u32 11, "AxisHandle"=w1106) -> ("AxisHandle"=w1105:u32)  [unwired: 1 in, 2 out]
          }
          frame #8 {
            n594 = Wait Until Next ms Multiple(millisecond multiple=u32 100 ("毫秒倍数")) -> ()  [unwired: 1 out]
          }
          frame #9 {
            n595 = while {
              tunnel: w1112 -> [w1115]
              tunnel: [w1114] -> w1111
              stop <- w1113 stop-if-true
              n596 = call <userlib>:"Acm_AxGetCmdVelocity.vi"("AxisHandle"=w1115) -> ("Velocity"=w1117:dbl, "AxisHandle"=w1114:u32)  [unwired: 1 in, 2 out]
              n597 = Wait Until Next ms Multiple(millisecond multiple=u32 50 ("毫秒倍数")) -> ()  [unwired: 1 out]
              n598 = Equal To 0?(x=w1117) -> (x = 0?=w1113:bool)
            }
          }
          frame #10 {
            n599 = call "PCI1220U角度置零.vi"("AxisHandle IN"=w1119) -> ("AxisHandle OUT"=w1118:u32)  [unwired: 10 in]
          }
          frame #11 {
            n600 = while {
              tunnel: w1121 -> [w1123]
              tunnel: [w1122] -> w1120
              stop <- w1126 stop-if-true
              n601 = Wait Until Next ms Multiple(millisecond multiple=u32 50 ("毫秒倍数")) -> ()  [unwired: 1 out]
              n602 = call "PCI1220U扭矩轴位置模式.vi"("Distance"=10.0, "AxisHandle IN"=w1123) -> ("AbsSuccess"=w1126:bool, "AxisHandle OUT"=w1122:u32)  [unwired: 8 in]
            }
          }
          frame #12 {
            n603 = Wait Until Next ms Multiple(millisecond multiple=u32 500 ("毫秒倍数")) -> ()  [unwired: 1 out]
          }
          frame #13 {
            n604 = while {
              tunnel: w1130 -> [w1133]
              tunnel: [w1132] -> w1129
              stop <- w1131 stop-if-true
              n605 = call <userlib>:"Acm_AxGetCmdVelocity.vi"("AxisHandle"=w1133) -> ("Velocity"=w1135:dbl, "AxisHandle"=w1132:u32)  [unwired: 1 in, 2 out]
              n606 = Wait Until Next ms Multiple(millisecond multiple=u32 50 ("毫秒倍数")) -> ()  [unwired: 1 out]
              n607 = Equal To 0?(x=w1135) -> (x = 0?=w1131:bool)
            }
          }
          frame #14 {
            n608 = call "PCI1220U角度置零.vi"("AxisHandle IN"=w1136) -> ()  [unwired: 10 in, 1 out]
          }
          frame #15 {
            n609 = while {
              tunnel: [w1140] -> w1137
              stop <- w1139 stop-if-true
              n610 = local read "电动缸电机"() -> (w1141:u32)
              n611 = Wait Until Next ms Multiple(millisecond multiple=u32 50 ("毫秒倍数")) -> ()  [unwired: 1 out]
              n612 = local read "齿条右极限"() -> (w1138:dbl)
              n613 = call "PCI1240电动缸位置模式 .vi"("Distance"=w1138, "AxisHandle IN"=w1141) -> ("AbsSuccess"=w1139:bool, "AxisHandle OUT"=w1140:u32)  [unwired: 8 in]
            }
          }
          frame #16 {
            n614 = while {
              tunnel: w1144 -> [w1152]
              tunnel: [w1150] -> w1143
              stop <- w1145 stop-if-true
              n615 = local read "齿条推拉力(N)"() -> (w1149:dbl)
              n616 = Wait Until Next ms Multiple(millisecond multiple=u32 50 ("毫秒倍数")) -> ()  [unwired: 1 out]
              n617 = call <userlib>:"Acm_AxGetCmdVelocity.vi"("AxisHandle"=w1152) -> ("Velocity"=w1153:dbl, "AxisHandle"=w1150:u32)  [unwired: 1 in, 2 out]
              n618 = Equal To 0?(x=w1153) -> (x = 0?=w1147:bool)
              n619 = Greater Or Equal?(x=w1149, y=300.0) -> (x >= y?=w1146:bool)
              n620 = Or(x=w1147, y=w1146) -> (x .or. y?=w1145:bool)
            }
          }
          frame #17 {
            n621 = while {
              tunnel: w1154 -> [w1158]
              tunnel: [w1157] -> _
              stop <- w1156 stop-if-true
              n622 = call "PCI1220U停止.vi"("AxisHandle IN"=w1158) -> ("完成"=w1156:bool, "AxisHandle OUT"=w1157:u32)  [unwired: 9 in]
              n623 = Wait (ms)(milliseconds to wait=u32 50 ("毫秒倍数")) -> ()  [unwired: 1 out]
            }
          }
          frame #18 {
            n624 = local write "工步号"(u32 100 ("工步号")) -> ()
          }
        }
      }
      frame 100 {
        n625 = flat-sequence {
          tunnel: [w1193] -> w1183
          tunnel: [w1191] -> w1182
          tunnel: [w1185] -> w1170
          tunnel: [w1184] -> w1167
          tunnel: w1183 -> [w1200]
          tunnel: w1182 -> [w1197]
          tunnel: ["F:\\报表存储\\" ("字符串")] -> w1181
          tunnel: w1170 -> [w1199]
          tunnel: [w1200] -> w1169
          tunnel: [w1199] -> w1168
          tunnel: w1167 -> [w1198]
          tunnel: [w1198] -> w1166
          tunnel: [w1197] -> w1165
          tunnel: w1181 -> [w1212]
          tunnel: [w1219] -> w1180
          tunnel: [w1217] -> w1179
          tunnel: [w1216] -> w1178
          tunnel: [w1215] -> w1177
          tunnel: w1169 -> [w1211]
          tunnel: w1168 -> [w1210]
          tunnel: w1166 -> [w1209]
          tunnel: w1165 -> [w1202]
          tunnel: [w1204] -> w1160
          tunnel: w1180 -> [w1226]
          tunnel: [w1227] -> w1176
          tunnel: w1179 -> [w1227]
          tunnel: w1178 -> [w1225]
          tunnel: w1177 -> [w1224]
          tunnel: [w1223] -> w1175
          tunnel: [w1222] -> w1174
          tunnel: [w1221] -> w1161
          tunnel: w1160 -> [w1221]
          tunnel: [w1234] -> w1173
          tunnel: w1176 -> [w1234]
          tunnel: w1175 -> [w1233]
          tunnel: [w1233] -> w1172
          tunnel: [w1232] -> w1171
          tunnel: w1174 -> [w1232]
          tunnel: [w1230] -> w1162
          tunnel: w1161 -> [w1230]
          tunnel: w1173 -> [w1237]
          tunnel: w1172 -> [w1245]
          tunnel: w1171 -> [w1244]
          tunnel: [w1236] -> w1163
          tunnel: w1162 -> [w1236]
          tunnel: [w1253] -> w1164
          tunnel: w1163 -> [w1253]
          tunnel: w1164 -> [w1255]
          frame #0 {
            n626 = local read "产品ID"() -> (w1192:string)
            n627 = Format Date/Time String(time format string (%c)="%Y%m%d" ("时间格式字符串(%c)")) -> (date/time string=w1186:string)  [unwired: 2 in]
            n628 = String Subset(string=w1186, offset (0)=6 ("偏移量(0)"), length (rest)=2 ("长度（剩余）")) -> (substring=w1184:string)
            n629 = String Subset(string=w1186, offset (0)=4 ("偏移量(0)"), length (rest)=2 ("长度（剩余）")) -> (substring=w1185:string)
            n630 = String Subset(string=w1186, offset (0)=0 ("偏移量(0)"), length (rest)=4 ("长度（剩余）")) -> (substring=w1193:string)
            n631 = call <vilib>:"Trim Whitespace.vi"("string"=w1192) -> ("trimmed string"=w1191:string)  [unwired: 1 in]
          }
          frame #1 {
          }
          frame #2 {
            w1203 = "\\" ("字符串")
            n632 = Concatenate Strings(w1212, w1211, w1203, w1210, w1203, w1209, w1203, w1202, w1203) -> (w1206:string)
            n633 = Concatenate Strings(w1212, w1211, w1203, w1210, w1203, w1209, w1203, w1202, w1203) -> (w1220:string)
            n634 = Concatenate Strings(w1206, w1202, "间隙曲线.JPG" ("字符串")) -> (w1218:string)
            n635 = Concatenate Strings(w1206, "轴向力曲线数组.txt" ("字符串")) -> (w1215:string)
            n636 = Concatenate Strings(w1206, "扭动曲线数组.txt" ("字符串")) -> (w1216:string)
            n637 = Concatenate Strings(w1206, w1202, "轴向力曲线.JPG" ("字符串")) -> (w1208:string)
            n638 = String To Path(string=w1218) -> (path=w1217:path)
            n639 = String To Path(string=w1220) -> (path=w1219:path)
            n640 = String To Path(string=w1208) -> (path=w1204:path)
          }
          frame #3 {
            n641 = call <vilib>:"Check if File or Folder Exists.vi"("path"=w1226) -> ("file or folder exists?"=w1228:bool)  [unwired: 8 in, 2 out]
            n642 = case shown="假" w1228 {
              tunnel: w1226 -> [w1229 _]
              frame False {
                n643 = Create Folder(path (use dialog)=w1229) -> ()  [unwired: 2 in, 3 out]
              }
              frame True {
              }
            }
            n644 = String To Path(string=w1224) -> (path=w1222:path)
            n645 = String To Path(string=w1225) -> (path=w1223:path)
          }
          frame #4 {
            n646 = local write "选项卡控件"(T1."间隙测量" ("选项卡控件")) -> ()
            n647 = Wait Until Next ms Multiple(millisecond multiple=u32 1000 ("毫秒倍数")) -> ()  [unwired: 1 out]
          }
          frame #5 {
            n648 = disable-structure shown="禁用" {
              disable-tunnel: w1237 -> [w1246 _]
              frame Disabled {
                w1250 = T2 2 items=["快速打印", "标准报表", "HTML", "双字节", "Excel"] ("report type (Quick Print)")
                w1249 = T3 1 items=["完整前面板", "前面板可见部分", "图标、说明、前面板和程序框图", "说明信息: 使用前面板", "说明信息: 作为子VI使用", "说明信息: 完整", "说明信息: 自定义"] ("contents (complete front panel)")
                n649 = Current VI's Path() -> (path=w1248:path)
                n650 = call-poly <vilib>:"Easy Print VI Panel or Documentation.vi"("report type (Quick Print)"=w1250, "contents (complete front panel)"=w1249, "VI path"=w1248) -> ("error out"=w1252:errorcluster, "report out"=w1251:refnum<class "NI_report.lvclass">)  [unwired: 1 in, 6 out]
                n651 = call-dynamic "Save Report to File.vi"("report in"=w1251, "report file path"=w1246, "error in (no error)"=w1252) -> ("error out"=→"error out 3":errorcluster)  [unwired: 2 in, 10 out]
              }
              frame Enabled {
              }
            }
            n652 = local read "间隙Y数组"() -> (w1242:dbl[])
            n653 = local read "间隙X数组"() -> (w1243:dbl[])
            n654 = local read "轴向力Y"() -> (w1240:dbl[])
            n655 = local read "轴向力X"() -> (w1241:dbl[])
            n656 = call "导出曲线数组.vi"("file path (dialog if empty)"=w1245, "数组 2"=w1242, "数组"=w1243) -> ()  [unwired: 9 in]
            n657 = call "导出曲线数组.vi"("file path (dialog if empty)"=w1244, "数组 2"=w1240, "数组"=w1241) -> ()  [unwired: 9 in]
            n658 = control-ref of="本VI"() -> (w1239:refnum<vi>)
            n659 = invoke class="VI" method="FP.Get Image"(reference=w1239) -> ("image data"=w1238:T4)  [unwired: 5 in, 5 out]
            n660 = call <vilib>:"Write JPEG File.vi"("image data"=w1238, "path to JPEG file"=w1237) -> ()  [unwired: 8 in, 2 out]
          }
          frame #6 {
            n661 = local write "选项卡控件"(T1."轴向力测量" ("选项卡控件")) -> ()
          }
          frame #7 {
            n662 = control-ref of="本VI"() -> (w1256:refnum<vi>)
            n663 = invoke class="VI" method="FP.Get Image"(reference=w1256) -> ("image data"=w1257:T4)  [unwired: 5 in, 5 out]
            n664 = call <vilib>:"Write JPEG File.vi"("image data"=w1257, "path to JPEG file"=w1255) -> ()  [unwired: 8 in, 2 out]
          }
          frame #8 {
            n665 = local read "联线按钮"() -> (w1258:bool)
            n666 = case shown="真" w1258 {
              frame False {
              }
              frame True {
                n667 = flat-sequence {
                  tunnel: [w1261] -> w1259
                  tunnel: [w1269] -> w1260
                  tunnel: w1259 -> [w1265]
                  tunnel: w1260 -> [w1283]
                  frame #0 {
                    n668 = local read "轴向力及全行程间隙合格"() -> (w1262:bool)
                    n669 = local read "单点间隙合格"() -> (w1263:bool)
                    n670 = And(x=w1263, y=w1262) -> (x .and. y?=w1261:bool)
                  }
                  frame #1 {
                    n671 = local read "左全行程间隙"() -> (w1272:dbl)
                    n672 = Boolean To (0,1)(Boolean=w1265) -> (0, 1=w1267:i16)
                    n673 = local read "中间位置间隙"() -> (w1275:dbl)
                    n674 = local read "员工ID"() -> (w1280:string)
                    n675 = local read "FGCS"() -> (w1277:string)
                    n676 = local read "KSJJ"() -> (w1279:string)
                    n677 = local read "产品ID"() -> (w1281:string)
                    n678 = Number To Decimal String(number=w1267, width (-)=i16 1 ("宽度(-)")) -> (decimal integer string=w1264:string)
                    n679 = Format Date/Time String(time format string (%c)="%Y%m%d%H%M" ("时间格式字符串(%c)")) -> (date/time string=w1278:string)  [unwired: 2 in]
                    n680 = Number To Fractional String(number=w1272, precision (6)=i16 3 ("精度(6)")) -> (F-format string=w1270:string)  [unwired: 2 in]
                    n681 = Number To Fractional String(number=w1275, precision (6)=i16 3 ("精度(6)")) -> (F-format string=w1271:string)  [unwired: 2 in]
                    n682 = Build Array(w1281, w1280, "1", w1264, w1279, w1278, w1277, "Q14073-11A", w1271, w1270) -> (w1269:string[])
                  }
                  frame #2 {
                    n683 = Wait (ms)(milliseconds to wait=u32 500 ("等待时间（毫秒）")) -> ()  [unwired: 1 out]
                    n684 = call "数据库更新.vi"("设备号"="06", "数据"=w1283) -> ()  [unwired: 13 in, 1 out]
                  }
                  frame #3 {
                  }
                }
              }
            }
          }
          frame #9 {
            n685 = local write "产品ID"("") -> ()
            n686 = local write "工步号"(u32 0 ("工步号")) -> ()
          }
        }
      }
    }
    n687 = Wait (ms)(milliseconds to wait=u32 50 ("毫秒倍数")) -> ()  [unwired: 1 out]
    n688 = local read "停止"() -> (w7:bool)
  }
  n689 = while {
    stop <- w1288 stop-if-true
    n690 = event shown="[2] \"参数修改\": 值改变" {
      selector: _ -> [_ _ _ _ _ _ _]
      dyn-events: _ -> [_ _ _ _ _ _ _]
      timeout: 500 -> [_ _ _ _ _ _ _]
      event Timeout {
        n691 = event-data() -> ()  [unwired: 3 out]
      }
      event "停止": Value Change {
        n692 = event-data() -> ()  [unwired: 6 out]
        n693 = flat-sequence {
          frame #0 {
            n694 = Wait (ms)(milliseconds to wait=u32 1000 ("毫秒倍数")) -> ()  [unwired: 1 out]
          }
          frame #1 {
            n695 = Quit LabVIEW(quit? (T)=TRUE ("停止？(T)")) -> ()
          }
        }
      }
      event "参数修改": Value Change {
        n696 = event-data() -> ()  [unwired: 6 out]
        n697 = while {
          i -> [w1295]
          stop <- w1294 stop-if-true
          n698 = local read "型号数量"() -> (w1296:i32)
          n699 = local read "参数浏览表"() -> (w1297:string[][])
          n700 = Wait Until Next ms Multiple(millisecond multiple=u32 50 ("毫秒倍数")) -> ()  [unwired: 1 out]
          n701 = Greater Or Equal?(x=w1295, y=w1296) -> (x >= y?=w1294:bool)
          n702 = Index Array(array=w1297, index (col)=w1295) -> (element=w1293:string[])  [unwired: 1 in]
          n703 = stacked-sequence {
            tunnel: w1293 -> [w1333]
            frame #0 {
              n704 = Index Array(array=w1333, index #1=0 ("索引"), index #2=2 ("索引"), index #3=3 ("索引"), index #4=4 ("索引"), index #5=5 ("索引"), index #6=6 ("索引"), index #7=7 ("索引"), index #8=8 ("索引"), index #9=9 ("索引"), index #10=10 ("索引"), index #11=11 ("索引"), index #12=12 ("索引"), index #13=13 ("索引"), index #14=14 ("索引"), index #15=15 ("索引"), index #16=16 ("索引"), index #17=17 ("索引"), index #18=18 ("索引"), index #19=19 ("索引"), index #20=20 ("索引")) -> (element #1=w1300:string, element #2=w1329:string, element #3=w1328:string, element #4=w1327:string, element #5=w1326:string, element #6=w1325:string, element #7=w1324:string, element #8=w1323:string, element #9=w1322:string, element #10=w1321:string, element #11=w1320:string, element #12=w1311:string, element #13=w1310:string, element #14=w1309:string, element #15=w1308:string, element #16=w1307:string, element #17=w1306:string, element #18=w1303:string, element #19=w1302:string, element #20=w1299:string)
              n705 = call "创建文本"("测头机构轴移动速度"=w1329, "测头机构轴检测位"=w1328, "测头机构轴待检位"=w1327, "测头机构轴后退位"=w1326, "齿条移动速度"=w1325, "齿条左极限"=w1324, "齿条右极限"=w1323, "旋转齿条轴找帽转速"=w1322, "旋转齿条轴测量转速"=w1321, "测量点扭矩"=w1320, "总行程最小值"=w1311, "总行程最大值"=w1310, "最大轴向力"=w1309, "轴向力波动"=w1308, "平均轴向力最小值"=w1307, "平均轴向力最大值"=w1306, "总圈数最小值"=w1303, "总圈数最大值"=w1302, "中间位置"=w1299, "产品型号"=w1300) -> ("Result"=w1319:string)  [unwired: 6 in, 1 out]
              n706 = local read "ADODB._Connection Out 2"() -> (w1318:refnum<k7>)
              n707 = call "SQL Execute.vi"("Command Text"=w1319, "ADODB._Connection In"=w1318) -> ("error out"=w1331:errorcluster, "ADODB._Connection Out"=w1332:refnum<k7>)  [unwired: 6 in, 2 out]
              n708 = call "ADO Connection Close.vi"("error in (no error)"=w1331, "ADODB._Connection In"=w1332) -> ("error out"=→"error out":errorcluster)  [unwired: 8 in, 1 out]
            }
          }
        }
      }
      event "参数查询": Value Change {
        n709 = event-data() -> ()  [unwired: 6 out]
        n710 = flat-sequence {
          tunnel: [w1356] -> w1349
          tunnel: [w1355] -> w1348
          tunnel: [w1354] -> w1345
          tunnel: w1349 -> [w1360]
          tunnel: w1348 -> [w1362]
          tunnel: [w1362] -> w1347
          tunnel: [w1361] -> w1346
          tunnel: w1345 -> [w1361]
          tunnel: w1347 -> [_]
          tunnel: w1346 -> [_]
          frame #0 {
            n711 = call-poly <vilib>:"Read From Spreadsheet File.vi"("file path (dialog if empty)"=path "D:/Q14070-Z060人机界面/参数/参数项.txt") -> ("first row"=w1350:string[])  [unwired: 6 in, 4 out]
            n712 = property on="参数浏览表" class="Tbl (严格)"("Row Headers[]"=w1350) -> ()  [unwired: 2 in, 2 out]
          }
          frame #1 {
            n713 = local read "ADODB._Connection Out 2"() -> (w1353:refnum<k7>)
            n714 = call "SQL Execute.vi"("Command Text"="SELECT * FROM 测试参数表;", "ADODB._Connection In"=w1353) -> ("error out"=w1354:errorcluster, "Data"=w1358:string[][], "ADODB._Connection Out"=w1355:refnum<k7>)  [unwired: 6 in, 1 out]
            n715 = Transpose 2D Array(2D array=w1358) -> (transposed array=w1356:string[][])
            n716 = Index Array(array=w1356, index (row)=0 ("索引 (行)")) -> (element=w1357:string[])  [unwired: 1 in]
            n717 = property on="参数浏览表" class="Tbl (严格)"("Column Headers[]"=w1357) -> ()  [unwired: 2 in, 2 out]
          }
          frame #2 {
            n718 = local write "参数浏览表"(w1360) -> ()
          }
          frame #3 {
          }
        }
      }
      event "传感器参数保存": Value Change {
        n719 = event-data() -> ()  [unwired: 6 out]
        n720 = flat-sequence {
          tunnel: [w1388] -> w1385
          tunnel: [w1387] -> w1384
          tunnel: [w1386] -> w1383
          tunnel: [w1394] -> w1382
          tunnel: w1385 -> [w1394]
          tunnel: [w1393] -> w1381
          tunnel: w1384 -> [w1393]
          tunnel: [w1392] -> w1380
          tunnel: w1383 -> [w1392]
          tunnel: [w1391] -> w1379
          tunnel: [w1390] -> w1378
          tunnel: [w1389] -> w1377
          tunnel: [w1395] -> w1376
          tunnel: [w1401] -> w1375
          tunnel: w1382 -> [w1401]
          tunnel: [w1400] -> w1374
          tunnel: w1381 -> [w1400]
          tunnel: w1380 -> [w1399]
          tunnel: [w1399] -> w1373
          tunnel: [w1398] -> w1372
          tunnel: w1379 -> [w1398]
          tunnel: [w1397] -> w1371
          tunnel: w1378 -> [w1397]
          tunnel: [w1396] -> w1370
          tunnel: w1377 -> [w1396]
          tunnel: w1376 -> [w1420]
          tunnel: [w1420] -> w1369
          tunnel: w1375 -> [w1419]
          tunnel: w1374 -> [w1412]
          tunnel: w1373 -> [w1411]
          tunnel: w1372 -> [w1405]
          tunnel: w1371 -> [w1404]
          tunnel: w1370 -> [w1410]
          tunnel: [w1409] -> w1368
          tunnel: [w1408] -> w1367
          tunnel: [w1407] -> w1366
          tunnel: [w1403] -> w1365
          tunnel: [w1402] -> w1364
          tunnel: [w1406] -> w1363
          tunnel: w1369 -> [w1428]
          tunnel: w1368 -> [w1427]
          tunnel: w1367 -> [w1426]
          tunnel: w1366 -> [w1425]
          tunnel: w1365 -> [w1424]
          tunnel: w1364 -> [w1423]
          tunnel: w1363 -> [w1422]
          frame #0 {
            n721 = local read "齿条推拉力零点偏移"() -> (w1387:dbl)
            n722 = local read "间隙位移零点偏移"() -> (w1388:dbl)
            n723 = local read "齿条扭矩零点偏移"() -> (w1386:dbl)
          }
          frame #1 {
            n724 = local read "齿条推拉力比例偏移"() -> (w1390:dbl)
            n725 = local read "间隙位移比例偏移"() -> (w1391:dbl)
            n726 = local read "齿条扭矩比例偏移"() -> (w1389:dbl)
          }
          frame #2 {
            n727 = local read "ADODB._Connection Out 2"() -> (w1395:refnum<k7>)
          }
          frame #3 {
            n728 = Number To Fractional String(number=w1419, precision (6)=i16 2 ("精度(6)")) -> (F-format string=w1409:string)  [unwired: 2 in]
            n729 = Number To Fractional String(number=w1411, precision (6)=i16 2 ("精度(6)")) -> (F-format string=w1407:string)  [unwired: 2 in]
            n730 = Number To Fractional String(number=w1410, precision (6)=i16 2 ("精度(6)")) -> (F-format string=w1406:string)  [unwired: 2 in]
            n731 = Number To Fractional String(number=w1412, precision (6)=i16 2 ("精度(6)")) -> (F-format string=w1408:string)  [unwired: 2 in]
            n732 = Number To Fractional String(number=w1405, precision (6)=i16 2 ("精度(6)")) -> (F-format string=w1403:string)  [unwired: 2 in]
            n733 = Number To Fractional String(number=w1404, precision (6)=i16 2 ("精度(6)")) -> (F-format string=w1402:string)  [unwired: 2 in]
          }
          frame #4 {
            n734 = call "创建文本3"("4"=w1424, "6"=w1422, "1"=w1427, "2"=w1426, "3"=w1425, "5"=w1423) -> ("Result"=w1429:string)  [unwired: 8 in, 1 out]
            n735 = call "SQL Execute.vi"("Command Text"=w1429, "ADODB._Connection In"=w1428) -> ("error out"=→"error out 4":errorcluster)  [unwired: 6 in, 3 out]
          }
        }
      }
      event "产品ID": Value Change {
        n736 = event-data() -> ()  [unwired: 7 out]
        n737 = Format Date/Time String(time format string (%c)="%Y%m%d%H%M" ("时间格式字符串(%c)")) -> (date/time string=w1430:string)  [unwired: 2 in]
        n738 = local write "KSJJ"(w1430) -> ()
      }
      event "电动缸回零": Mouse Down {
        n739 = event-data() -> ()  [unwired: 6 out]
        n740 = stacked-sequence {
          frame #0 {
            n741 = flat-sequence {
              tunnel: [w1448] -> w1437
              tunnel: [w1441] -> w1434
              tunnel: w1437 -> [w1451]
              tunnel: [w1451] -> w1436
              tunnel: [w1449] -> w1435
              tunnel: w1434 -> [w1449]
              tunnel: w1436 -> [w1453]
              tunnel: [w1453] -> w1438
              tunnel: w1435 -> [w1452]
              tunnel: [w1452] -> w1433
              tunnel: w1438 -> [w1463]
              tunnel: w1433 -> [w1462]
              frame #0 {
                n742 = local write "电动缸速度(mm/s)"(15.0 ("电动缸速度(mm/s)")) -> ()
                n743 = local write "测头机构轴速度(mm/s)"(10.0 ("电动缸速度(mm/s)")) -> ()
              }
              frame #1 {
                n744 = local read "测头机构电机"() -> (w1445:u32)
                n745 = local read "电动缸电机"() -> (w1442:u32)
                n746 = call <userlib>:"Acm_AxHome.vi"("DirMode"=u32 0, "HomeMode"=u32 11, "AxisHandle"=w1445) -> ("AxisHandle"=w1448:u32)  [unwired: 1 in, 2 out]
                n747 = call <userlib>:"Acm_AxHome.vi"("DirMode"=u32 1, "HomeMode"=u32 11, "AxisHandle"=w1442) -> ("AxisHandle"=w1441:u32)  [unwired: 1 in, 2 out]
              }
              frame #2 {
                n748 = Wait Until Next ms Multiple(millisecond multiple=u32 100 ("毫秒倍数")) -> ()  [unwired: 1 out]
              }
              frame #3 {
                n749 = while {
                  tunnel: w1453 -> [w1461]
                  stop <- w1459 stop-if-true
                  n750 = call <userlib>:"Acm_AxGetCmdVelocity.vi"("AxisHandle"=w1461) -> ("Velocity"=w1460:dbl)  [unwired: 1 in, 3 out]
                  n751 = Wait Until Next ms Multiple(millisecond multiple=u32 50 ("毫秒倍数")) -> ()  [unwired: 1 out]
                  n752 = Equal To 0?(x=w1460) -> (x = 0?=w1459:bool)
                }
                n753 = while {
                  tunnel: w1452 -> [w1457]
                  stop <- w1455 stop-if-true
                  n754 = call <userlib>:"Acm_AxGetCmdVelocity.vi"("AxisHandle"=w1457) -> ("Velocity"=w1456:dbl)  [unwired: 1 in, 3 out]
                  n755 = Wait Until Next ms Multiple(millisecond multiple=u32 50 ("毫秒倍数")) -> ()  [unwired: 1 out]
                  n756 = Equal To 0?(x=w1456) -> (x = 0?=w1455:bool)
                }
              }
              frame #4 {
                n757 = call "PCI1220U角度置零.vi"("AxisHandle IN"=w1463) -> ()  [unwired: 10 in, 1 out]
                n758 = call "PCI1220U角度置零.vi"("AxisHandle IN"=w1462) -> ()  [unwired: 10 in, 1 out]
              }
              frame #5 {
              }
              frame #6 {
              }
            }
          }
          frame #1 {
            n759 = flat-sequence {
              tunnel: [w1475] -> w1470
              tunnel: w1470 -> [w1477]
              tunnel: [w1477] -> w1469
              tunnel: w1469 -> [w1478]
              tunnel: [w1478] -> w1468
              tunnel: w1468 -> [w1484]
              tunnel: [w1483] -> w1465
              tunnel: w1465 -> [w1486]
              tunnel: [w1486] -> w1464
              tunnel: w1464 -> [w1488]
              tunnel: [w1487] -> w1467
              tunnel: w1467 -> [w1494]
              tunnel: [w1494] -> w1466
              tunnel: w1466 -> [w1499]
              frame #0 {
                n760 = local write "旋转齿条轴速度(°/s)"(5.0 ("电动缸速度(mm/s)")) -> ()
              }
              frame #1 {
                n761 = local read "旋转齿条电机"() -> (w1472:u32)
                n762 = call <userlib>:"Acm_AxHome.vi"("DirMode"=u32 0, "HomeMode"=u32 11, "AxisHandle"=w1472) -> ("AxisHandle"=w1475:u32)  [unwired: 1 in, 2 out]
              }
              frame #2 {
                n763 = Wait Until Next ms Multiple(millisecond multiple=u32 100 ("毫秒倍数")) -> ()  [unwired: 1 out]
              }
              frame #3 {
                n764 = while {
                  tunnel: w1478 -> [w1482]
                  stop <- w1480 stop-if-true
                  n765 = call <userlib>:"Acm_AxGetCmdVelocity.vi"("AxisHandle"=w1482) -> ("Velocity"=w1481:dbl)  [unwired: 1 in, 3 out]
                  n766 = Wait Until Next ms Multiple(millisecond multiple=u32 50 ("毫秒倍数")) -> ()  [unwired: 1 out]
                  n767 = Equal To 0?(x=w1481) -> (x = 0?=w1480:bool)
                }
              }
              frame #4 {
                n768 = call "PCI1220U角度置零.vi"("AxisHandle IN"=w1484) -> ("AxisHandle OUT"=w1483:u32)  [unwired: 10 in]
              }
              frame #5 {
                n769 = Wait (ms)(milliseconds to wait=u32 100 ("等待时间（毫秒）")) -> ()  [unwired: 1 out]
              }
              frame #6 {
                n770 = while {
                  tunnel: [w1492] -> w1487
                  tunnel: w1488 -> [w1489]
                  stop <- w1491 stop-if-true
                  n771 = Wait Until Next ms Multiple(millisecond multiple=u32 50 ("毫秒倍数")) -> ()  [unwired: 1 out]
                  n772 = call "PCI1220U扭矩轴位置模式.vi"("Distance"=10.0, "AxisHandle IN"=w1489) -> ("AbsSuccess"=w1491:bool, "AxisHandle OUT"=w1492:u32)  [unwired: 8 in]
                }
              }
              frame #7 {
                n773 = while {
                  tunnel: w1494 -> [w1497]
                  stop <- w1495 stop-if-true
                  n774 = call <userlib>:"Acm_AxGetCmdVelocity.vi"("AxisHandle"=w1497) -> ("Velocity"=w1498:dbl)  [unwired: 1 in, 3 out]
                  n775 = Wait Until Next ms Multiple(millisecond multiple=u32 50 ("毫秒倍数")) -> ()  [unwired: 1 out]
                  n776 = Equal To 0?(x=w1498) -> (x = 0?=w1495:bool)
                }
              }
              frame #8 {
                n777 = call "PCI1220U角度置零.vi"("AxisHandle IN"=w1499) -> ()  [unwired: 10 in, 1 out]
              }
            }
          }
          frame #2 {
            n778 = flat-sequence {
              frame #0 {
                n779 = while {
                  stop <- w1503 stop-if-true
                  n780 = local read "电动缸回零"() -> (w1504:bool)
                  n781 = local write "回零完成"(TRUE ("回零完成")) -> ()
                  n782 = local write "电动缸回零"(FALSE ("电动缸回零")) -> ()
                  n783 = Wait Until Next ms Multiple(millisecond multiple=u32 50 ("毫秒倍数")) -> ()  [unwired: 1 out]
                  n784 = Not(x=w1504) -> (.not. x?=w1503:bool)
                }
              }
            }
          }
        }
        n785 = Wait Until Next ms Multiple(millisecond multiple=u32 50 ("毫秒倍数")) -> ()  [unwired: 1 out]
      }
    }
    n786 = Wait (ms)(milliseconds to wait=u32 50 ("毫秒倍数")) -> ()  [unwired: 1 out]
    n787 = local read "停止"() -> (w1288:bool)
  }
  n788 = call "PCI1240电动缸位置模式 .vi"() -> ()  [unwired: 10 in, 2 out]
  n789 = while {
    stop <- w1506 stop-if-true
    n790 = stacked-sequence {
      frame #0 {
        n791 = flat-sequence {
          frame #0 {
          }
          frame #1 {
          }
          frame #2 {
            n792 = First Call?() -> (First Call?: T/F=w1507:bool)
            n793 = case shown="真" w1507 {
              frame False {
              }
              frame True {
                n794 = call "员工管理测试程序.vi"() -> ("员工姓名"=w1509:string, "员工ID"=w1508:string)  [unwired: 10 in]
                n795 = local write "员工ID"(w1508) -> ()
                n796 = local write "员工姓名"(w1509) -> ()
              }
            }
          }
          frame #3 {
          }
          frame #4 {
          }
          frame #5 {
          }
          frame #6 {
          }
        }
      }
      frame #1 {
        n797 = flat-sequence {
          frame #0 {
            n798 = property on="型号选择" class="Ring (严格)"() -> ("RingText.Text"=w1510:string)  [unwired: 2 in, 2 out]
            n799 = case shown="\"J706\"" w1510 {
              frame "J709", Default {
                w1511 = FALSE ("可见")
                w1512 = TRUE ("可见")
                n800 = property on="右180°内全行程间隙" class="DigNum (严格)"("Visible"=w1511) -> ()  [unwired: 2 in, 2 out]
                n801 = property on="右180°外全行程间隙" class="DigNum (严格)"("Visible"=w1511) -> ()  [unwired: 2 in, 2 out]
                n802 = property on="左180°外全行程间隙" class="DigNum (严格)"("Visible"=w1511) -> ()  [unwired: 2 in, 2 out]
                n803 = property on="左180°内全行程间隙" class="DigNum (严格)"("Visible"=w1511) -> ()  [unwired: 2 in, 2 out]
                n804 = property on="右全行程间隙" class="DigNum (严格)"("Visible"=w1512) -> ()  [unwired: 2 in, 2 out]
                n805 = property on="左全行程间隙" class="DigNum (严格)"("Visible"=w1512) -> ()  [unwired: 2 in, 2 out]
              }
              frame "J706" {
                w1513 = TRUE ("可见")
                w1514 = FALSE ("可见")
                n806 = property on="右180°内全行程间隙" class="DigNum (严格)"("Visible"=w1513) -> ()  [unwired: 2 in, 2 out]
                n807 = property on="右180°外全行程间隙" class="DigNum (严格)"("Visible"=w1513) -> ()  [unwired: 2 in, 2 out]
                n808 = property on="左180°外全行程间隙" class="DigNum (严格)"("Visible"=w1513) -> ()  [unwired: 2 in, 2 out]
                n809 = property on="左180°内全行程间隙" class="DigNum (严格)"("Visible"=w1513) -> ()  [unwired: 2 in, 2 out]
                n810 = property on="右全行程间隙" class="DigNum (严格)"("Visible"=w1514) -> ()  [unwired: 2 in, 2 out]
                n811 = property on="左全行程间隙" class="DigNum (严格)"("Visible"=w1514) -> ()  [unwired: 2 in, 2 out]
              }
            }
          }
          frame #1 {
            (unwired) string[] ["I急停按钮", "I自动旋钮", "I启动按钮", "I备用按钮", "I复位按钮", "I上阻挡器放行", "I下阻挡器放行", "I进支线按钮"] ("I0说明")
            (unwired) string[] ["I出支线按钮", "I主线顶升按钮", "I主线下降按钮", "I支线顶升按钮", "I支线下降按钮", "I气压报警", "未使用", "未使用"] ("I0说明")
            n812 = local read "间隙位移(mm)"() -> (w1517:dbl)
            n813 = Greater Or Equal?(x=w1517, y=4.0) -> (x >= y?=w1515:bool)
            n814 = case shown="真" w1515 {
              frame False {
              }
              frame True {
                n815 = local write "测头机构轴使能"(FALSE ("测头机构轴使能")) -> ()
              }
            }
          }
          frame #2 {
            (unwired) string[] ["I电动缸SRDY", "I电动缸ZSPD", "I电动缸ALRM", "I间隙进给SRDY", "I间隙进给ZSPD", "I间隙进给ALRM", "I间隙旋转SRPD", "I间隙旋转ZSPD"] ("I0说明")
            n816 = local read "测头机构轴位置(mm)"() -> (w1521:dbl)
            n817 = Greater Or Equal?(x=w1521, y=90.0) -> (x >= y?=w1519:bool)
            n818 = case shown="假" w1519 {
              frame False {
                w1522 = T5."Enabled" ("禁用")
                n819 = property on="测头气缸右移" class="Bool"("DisabledEnum"=w1522) -> ()  [unwired: 2 in, 2 out]
                n820 = property on="测头气缸左移" class="Bool"("DisabledEnum"=w1522) -> ()  [unwired: 2 in, 2 out]
                n821 = property on="测头气缸右移" class="Bool (严格)"("DisabledEnum"=w1522) -> ()  [unwired: 2 in, 2 out]
                n822 = property on="测头气缸左移" class="Bool (严格)"("DisabledEnum"=w1522) -> ()  [unwired: 2 in, 2 out]
              }
              frame True {
                w1523 = T5."Disabled" ("禁用")
                w1524 = FALSE ("测头气缸右移")
                n823 = local write "测头气缸右移"(w1524) -> ()
                n824 = local write "测头气缸左移"(w1524) -> ()
                n825 = property on="测头气缸右移" class="Bool"("DisabledEnum"=w1523) -> ()  [unwired: 2 in, 2 out]
                n826 = property on="测头气缸左移" class="Bool"("DisabledEnum"=w1523) -> ()  [unwired: 2 in, 2 out]
                n827 = property on="测头气缸右移" class="Bool (严格)"("DisabledEnum"=w1523) -> ()  [unwired: 2 in, 2 out]
                n828 = property on="测头气缸左移" class="Bool (严格)"("DisabledEnum"=w1523) -> ()  [unwired: 2 in, 2 out]
              }
            }
          }
          frame #3 {
            (unwired) string[] ["I间隙旋转ALRM", "I扭矩旋转SRPD", "I扭矩旋转ZSPD", "I扭矩旋转ALRM", "I拧紧机合格", "I拧紧机不合格", "I拧紧机报警", "未使用"] ("I0说明")
          }
        }
      }
      frame #2 {
        n829 = flat-sequence {
          frame #0 {
            (unwired) string[] ["I自制气缸进位", "I自制气缸原位", "I上工位检测", "I本工位检测", "I下工位检测", "I主线顶升上位", "I主线顶升下位", "I支线顶升上位"] ("I0说明")
          }
          frame #1 {
            (unwired) string[] ["I支线顶升下位", "I支线进到位", "I支线退到位", "I位移气缸原位", "I位移气缸进位", "I拧紧机在位", "I电动缸原位", "I电动缸进位"] ("I0说明")
          }
          frame #2 {
            (unwired) string[] ["未使用", "未使用", "未使用", "未使用", "未使用", "未使用", "未使用", "未使用"] ("I0说明")
          }
          frame #3 {
            (unwired) string[] ["未使用", "未使用", "未使用", "未使用", "未使用", "未使用", "未使用", "未使用"] ("I0说明")
          }
        }
        n830 = local read "本测试状态"() -> (w1526:bool)
        n831 = local read "本自动状态"() -> (w1527:bool)
        n832 = local read "本备料状态"() -> (w1525:bool)
        n833 = local write "本测试状态H"(w1526) -> ()
        n834 = local write "本自动状态H"(w1527) -> ()
        n835 = local write "本备料状态H"(w1525) -> ()
      }
      frame #3 {
        n836 = local read "报警工步号"() -> (w1529:dbl)
        n837 = local read "工步号"() -> (w1531:u32)
        n838 = case shown="50" w1531 {
          tunnel: [w1541 "请取胶瓶" ("工步描述") "请对锁紧螺母加力" ("工步描述") "灵敏度测试中" ("工步描述") "有油刚度测试中" ("工步描述") "安装好锁紧螺母后，按顶升按钮，夹具夹紧" ("工步描述") "请点击启动按钮进行试验" ("工步描述") "探头气缸右移" ("工步描述") "电动缸前进找中" ("工步描述") "探头前进测试开始" ("工步描述") "探头退回" ("工步描述") "轴向力测试中" ("工步描述") "测头后退夹抓松开" ("工步描述") "伺服回零" ("工步描述") "力特性试验完成" ("工步描述") "套好输出轴把手，按启动按钮，做回正力试验" ("工步描述") "回正力试验中" ("工步描述") "试验完成，将把手拉回，取下油管，按顶升按钮" ("工步描述") "拆下锁紧螺母和输入轴万向节，按顶升按钮" ("工步描述")] -> w1530
          frame 0, Default {
            n839 = local read "联线按钮"() -> (w1540:bool)
            n840 = case shown="真" w1540 {
              tunnel: ["等待工件" ("工步描述") "等待扫描条码" ("工步描述")] -> w1541
              frame False {
              }
              frame True {
              }
            }
          }
          frame 1 {
          }
          frame 2 {
          }
          frame 3 {
          }
          frame 4 {
          }
          frame 5 {
          }
          frame 6 {
          }
          frame 10 {
          }
          frame 15 {
          }
          frame 20 {
          }
          frame 30 {
          }
          frame 40 {
          }
          frame 45 {
          }
          frame 50 {
          }
          frame 55 {
          }
          frame 60 {
          }
          frame 70 {
          }
          frame 80 {
          }
          frame 56 {
          }
        }
        "工步提示" <- w1530
        n841 = case shown="3" w1529 {
          tunnel: [_ "操作步骤错请取胶瓶" "操作步骤错误请点标" "测头气缸不在原位" "急停被按下" "气压报警" "电动缸伺服报警" "旋转伺服服报警" "测头伺服服报警"] -> w1528
          frame 0, Default {
          }
          frame 1 {
          }
          frame 3 {
          }
          frame 2 {
          }
          frame 4 {
          }
          frame 5 {
          }
          frame 6 {
          }
          frame 7 {
          }
          frame 8 {
          }
        }
        "报警提示" <- w1528
      }
      frame #4 {
        n842 = local read "急停"() -> (w1562:bool)
        n843 = local read "红灯"() -> (w1564:bool)
        n844 = local read "复位"() -> (w1565:bool)
        n845 = local read "复位"() -> (w1567:bool)
        n846 = local read "红灯"() -> (w1566:bool)
        n847 = case shown="假" w1562 {
          frame False {
            w1570 = TRUE ("红灯")
            n848 = local write "红灯"(w1570) -> ()
            n849 = local write "复位"(w1570) -> ()
          }
          frame True {
            w1571 = FALSE ("复位")
            n850 = local write "红灯"(w1571) -> ()
            n851 = local write "复位"(w1571) -> ()
          }
        }
        n852 = Or(x=w1564, y=w1565) -> (x .or. y?=w1563:bool)
        n853 = case shown="真" w1563 {
          frame False {
          }
          frame True {
            n854 = local write "回零完成"(FALSE ("夹头夹紧控制")) -> ()
          }
        }
        n855 = local read "停止"() -> (w1569:bool)
        n856 = Compound Arithmetic op=OR(w1567, w1569, w1566) -> (w1568:bool)
        n857 = case shown="真" w1568 {
          frame False {
          }
          frame True {
            n858 = local read "测头机构电机"() -> (w1573:u32)
            n859 = local read "旋转齿条电机"() -> (w1574:u32)
            n860 = local read "电动缸电机"() -> (w1575:u32)
            n861 = call "PCI1220U停止.vi"("AxisHandle IN"=w1574) -> ()  [unwired: 9 in, 2 out]
            n862 = call "PCI1220U停止.vi"("AxisHandle IN"=w1575) -> ()  [unwired: 9 in, 2 out]
            n863 = call "PCI1220U停止.vi"("AxisHandle IN"=w1573) -> ()  [unwired: 9 in, 2 out]
          }
        }
      }
      frame #5 {
        n864 = local read "齿条扭矩(Nm)"() -> (w1578:dbl)
        n865 = local read "黄灯"() -> (w1576:bool)
        n866 = local read "旋转齿条轴左转"() -> (w1584:bool)
        n867 = Absolute Value(x=w1578) -> (abs(x)=w1583:dbl)
        n868 = local read "旋转齿条轴右转"() -> (w1579:bool)
        n869 = Not(x=w1584) -> (.not. x?=w1580:bool)
        n870 = Less?(x=w1583, y=20.0) -> (x < y?=w1581:bool)
        n871 = Compound Arithmetic op=AND(w1579, w1580, w1581, w1576) -> (w1577:bool)
        n872 = case shown="真" w1577 {
          frame False {
          }
          frame True {
            n873 = flat-sequence {
              tunnel: [w1588] -> w1586
              tunnel: w1586 -> [w1590]
              tunnel: [w1590] -> w1585
              tunnel: w1585 -> [w1601]
              frame #0 {
                n874 = local read "旋转齿条电机"() -> (w1587:u32)
                n875 = call "PCI1220U运行.vi"("方向"=enum32{"Negative", "Positive"}."Negative" ("Direction"), "AxisHandle IN"=w1587) -> ("AxisHandle OUT"=w1588:u32)  [unwired: 9 in]
              }
              frame #1 {
                n876 = while {
                  stop <- w1594 stop-if-true
                  n877 = Wait (ms)(milliseconds to wait=u32 50 ("毫秒倍数")) -> ()  [unwired: 1 out]
                  n878 = local read "齿条扭矩(Nm)"() -> (w1599:dbl)
                  n879 = local read "旋转齿条轴右转"() -> (w1596:bool)
                  n880 = local read "红灯"() -> (w1591:bool)
                  n881 = local read "复位"() -> (w1592:bool)
                  n882 = Absolute Value(x=w1599) -> (abs(x)=w1598:dbl)
                  n883 = Not(x=w1596) -> (.not. x?=w1593:bool)
                  n884 = Greater?(x=w1598, y=10.0) -> (0:w1595:bool)
                  n885 = Compound Arithmetic op=OR(w1595, w1593, w1592, w1591) -> (w1594:bool)
                }
              }
              frame #2 {
                n886 = call "PCI1220U停止.vi"("AxisHandle IN"=w1601) -> ()  [unwired: 9 in, 2 out]
              }
            }
          }
        }
      }
      frame #6 {
        n887 = local read "齿条扭矩(Nm)"() -> (w1606:dbl)
        n888 = local read "旋转齿条轴右转"() -> (w1610:bool)
        n889 = Absolute Value(x=w1606) -> (abs(x)=w1605:dbl)
        n890 = local read "旋转齿条轴左转"() -> (w1608:bool)
        n891 = local read "黄灯"() -> (w1602:bool)
        n892 = Not(x=w1610) -> (.not. x?=w1607:bool)
        n893 = Less?(x=w1605, y=20.0) -> (x < y?=w1603:bool)
        n894 = Compound Arithmetic op=AND(w1608, w1607, w1603, w1602) -> (w1609:bool)
        n895 = case shown="真" w1609 {
          frame False {
          }
          frame True {
            n896 = flat-sequence {
              tunnel: [w1614] -> w1612
              tunnel: w1612 -> [w1616]
              tunnel: [w1616] -> w1611
              tunnel: w1611 -> [w1627]
              frame #0 {
                n897 = local read "旋转齿条电机"() -> (w1613:u32)
                n898 = call "PCI1220U运行.vi"("方向"=enum32{"Negative", "Positive"}."Positive" ("Direction"), "AxisHandle IN"=w1613) -> ("AxisHandle OUT"=w1614:u32)  [unwired: 9 in]
              }
              frame #1 {
                n899 = while {
                  stop <- w1619 stop-if-true
                  n900 = Wait (ms)(milliseconds to wait=u32 50 ("毫秒倍数")) -> ()  [unwired: 1 out]
                  n901 = local read "齿条扭矩(Nm)"() -> (w1625:dbl)
                  n902 = local read "旋转齿条轴左转"() -> (w1622:bool)
                  n903 = local read "红灯"() -> (w1617:bool)
                  n904 = local read "复位"() -> (w1618:bool)
                  n905 = Absolute Value(x=w1625) -> (abs(x)=w1624:dbl)
                  n906 = Not(x=w1622) -> (.not. x?=w1620:bool)
                  n907 = Greater?(x=w1624, y=10.0) -> (0:w1621:bool)
                  n908 = Compound Arithmetic op=OR(w1618, w1617, w1621, w1620) -> (w1619:bool)
                }
              }
              frame #2 {
                n909 = call "PCI1220U停止.vi"("AxisHandle IN"=w1627) -> ()  [unwired: 9 in, 2 out]
              }
            }
          }
        }
      }
      frame #7 {
        n910 = local read "齿条推拉力(N)"() -> (w1632:dbl)
        n911 = local read "电动缸前进"() -> (w1629:bool)
        n912 = local read "电动缸后退"() -> (w1628:bool)
        n913 = Absolute Value(x=w1632) -> (abs(x)=w1636:dbl)
        n914 = local read "黄灯"() -> (w1630:bool)
        n915 = Not(x=w1628) -> (.not. x?=w1633:bool)
        n916 = Less?(x=w1636, y=1000.0) -> (x < y?=w1634:bool)
        n917 = Compound Arithmetic op=AND(w1629, w1633, w1630, w1634) -> (w1631:bool)
        n918 = case shown="真" w1631 {
          frame False {
          }
          frame True {
            n919 = flat-sequence {
              tunnel: [w1640] -> w1638
              tunnel: w1638 -> [w1642]
              tunnel: [w1642] -> w1637
              tunnel: w1637 -> [w1653]
              frame #0 {
                n920 = local read "电动缸电机"() -> (w1639:u32)
                n921 = call "PCI1220U运行.vi"("方向"=enum32{"Negative", "Positive"}."Positive" ("Direction"), "AxisHandle IN"=w1639) -> ("AxisHandle OUT"=w1640:u32)  [unwired: 9 in]
              }
              frame #1 {
                n922 = while {
                  stop <- w1650 stop-if-true
                  n923 = local read "电动缸前进"() -> (w1647:bool)
                  n924 = local read "齿条推拉力(N)"() -> (w1644:dbl)
                  n925 = Wait (ms)(milliseconds to wait=u32 50 ("毫秒倍数")) -> ()  [unwired: 1 out]
                  n926 = Absolute Value(x=w1644) -> (abs(x)=w1646:dbl)
                  n927 = local read "红灯"() -> (w1648:bool)
                  n928 = local read "复位"() -> (w1649:bool)
                  n929 = Greater?(x=w1646, y=1000.0) -> (0:w1643:bool)
                  n930 = Not(x=w1647) -> (.not. x?=w1651:bool)
                  n931 = Compound Arithmetic op=OR(w1649, w1648, w1651, w1643) -> (w1650:bool)
                }
              }
              frame #2 {
                n932 = call "PCI1220U停止.vi"("AxisHandle IN"=w1653) -> ()  [unwired: 9 in, 2 out]
              }
            }
          }
        }
      }
      frame #8 {
        n933 = local read "电动缸前进"() -> (w1654:bool)
        n934 = local read "齿条推拉力(N)"() -> (w1658:dbl)
        n935 = local read "电动缸后退"() -> (w1655:bool)
        n936 = Absolute Value(x=w1658) -> (abs(x)=w1662:dbl)
        n937 = local read "黄灯"() -> (w1656:bool)
        n938 = Not(x=w1654) -> (.not. x?=w1659:bool)
        n939 = Less?(x=w1662, y=1000.0) -> (x < y?=w1660:bool)
        n940 = Compound Arithmetic op=AND(w1655, w1659, w1656, w1660) -> (w1657:bool)
        n941 = case shown="真" w1657 {
          frame False {
          }
          frame True {
            n942 = flat-sequence {
              tunnel: [w1666] -> w1664
              tunnel: w1664 -> [w1668]
              tunnel: [w1668] -> w1663
              tunnel: w1663 -> [w1679]
              frame #0 {
                n943 = local read "电动缸电机"() -> (w1665:u32)
                n944 = call "PCI1220U运行.vi"("方向"=enum32{"Negative", "Positive"}."Negative" ("Direction"), "AxisHandle IN"=w1665) -> ("AxisHandle OUT"=w1666:u32)  [unwired: 9 in]
              }
              frame #1 {
                n945 = while {
                  stop <- w1676 stop-if-true
                  n946 = local read "电动缸后退"() -> (w1673:bool)
                  n947 = local read "齿条推拉力(N)"() -> (w1672:dbl)
                  n948 = Wait (ms)(milliseconds to wait=u32 50 ("毫秒倍数")) -> ()  [unwired: 1 out]
                  n949 = Absolute Value(x=w1672) -> (abs(x)=w1670:dbl)
                  n950 = local read "红灯"() -> (w1675:bool)
                  n951 = local read "复位"() -> (w1674:bool)
                  n952 = Greater?(x=w1670, y=1000.0) -> (0:w1669:bool)
                  n953 = Not(x=w1673) -> (.not. x?=w1677:bool)
                  n954 = Compound Arithmetic op=OR(w1674, w1675, w1677, w1669) -> (w1676:bool)
                }
              }
              frame #2 {
                n955 = call "PCI1220U停止.vi"("AxisHandle IN"=w1679) -> ()  [unwired: 9 in, 2 out]
              }
            }
          }
        }
      }
      frame #9 {
        n956 = local read "测头机构轴后退"() -> (w1680:bool)
        n957 = local read "测头机构轴前进"() -> (w1681:bool)
        n958 = local read "黄灯"() -> (w1682:bool)
        n959 = Not(x=w1680) -> (.not. x?=w1684:bool)
        n960 = Compound Arithmetic op=AND(w1681, w1684, w1682) -> (w1683:bool)
        n961 = case shown="真" w1683 {
          frame False {
          }
          frame True {
            n962 = flat-sequence {
              tunnel: [w1688] -> w1686
              tunnel: w1686 -> [w1690]
              tunnel: [w1690] -> w1685
              tunnel: w1685 -> [w1697]
              frame #0 {
                n963 = local read "测头机构电机"() -> (w1687:u32)
                n964 = call "PCI1220U运行.vi"("方向"=enum32{"Negative", "Positive"}."Positive" ("Direction"), "AxisHandle IN"=w1687) -> ("AxisHandle OUT"=w1688:u32)  [unwired: 9 in]
              }
              frame #1 {
                n965 = while {
                  stop <- w1694 stop-if-true
                  n966 = local read "测头机构轴前进"() -> (w1691:bool)
                  n967 = Wait (ms)(milliseconds to wait=u32 50 ("毫秒倍数")) -> ()  [unwired: 1 out]
                  n968 = local read "红灯"() -> (w1692:bool)
                  n969 = local read "复位"() -> (w1693:bool)
                  n970 = Not(x=w1691) -> (.not. x?=w1695:bool)
                  n971 = Compound Arithmetic op=OR(w1693, w1692, w1695) -> (w1694:bool)
                }
              }
              frame #2 {
                n972 = call "PCI1220U停止.vi"("AxisHandle IN"=w1697) -> ()  [unwired: 9 in, 2 out]
              }
            }
          }
        }
      }
      frame #10 {
        n973 = local read "测头机构轴前进"() -> (w1698:bool)
        n974 = local read "测头机构轴后退"() -> (w1699:bool)
        n975 = local read "黄灯"() -> (w1700:bool)
        n976 = Not(x=w1698) -> (.not. x?=w1702:bool)
        n977 = Compound Arithmetic op=AND(w1699, w1702, w1700) -> (w1701:bool)
        n978 = case shown="真" w1701 {
          frame False {
          }
          frame True {
            n979 = flat-sequence {
              tunnel: [w1706] -> w1704
              tunnel: w1704 -> [w1708]
              tunnel: [w1708] -> w1703
              tunnel: w1703 -> [w1715]
              frame #0 {
                n980 = local read "测头机构电机"() -> (w1705:u32)
                n981 = call "PCI1220U运行.vi"("方向"=enum32{"Negative", "Positive"}."Negative" ("Direction"), "AxisHandle IN"=w1705) -> ("AxisHandle OUT"=w1706:u32)  [unwired: 9 in]
              }
              frame #1 {
                n982 = while {
                  stop <- w1712 stop-if-true
                  n983 = local read "测头机构轴后退"() -> (w1709:bool)
                  n984 = Wait (ms)(milliseconds to wait=u32 50 ("毫秒倍数")) -> ()  [unwired: 1 out]
                  n985 = local read "红灯"() -> (w1711:bool)
                  n986 = local read "复位"() -> (w1710:bool)
                  n987 = Not(x=w1709) -> (.not. x?=w1713:bool)
                  n988 = Compound Arithmetic op=OR(w1710, w1711, w1713) -> (w1712:bool)
                }
              }
              frame #2 {
                n989 = call "PCI1220U停止.vi"("AxisHandle IN"=w1715) -> ()  [unwired: 9 in, 2 out]
              }
            }
          }
        }
      }
    }
    n990 = Wait (ms)(milliseconds to wait=u32 50 ("毫秒倍数")) -> ()  [unwired: 1 out]
    n991 = local read "停止"() -> (w1506:bool)
  }
  n992 = flat-sequence {
    tunnel: [w1719] -> w2
    tunnel: [w1717] -> w1
    tunnel: w2 -> [w1729]
    tunnel: w1 -> [w1728]
    frame #0 {
      n993 = First Call?() -> (First Call?: T/F=w1716:bool)
      n994 = case shown="真" w1716 {
        frame False {
        }
        frame True {
          n995 = while {
            i -> [w1724]
            stop <- w1722 stop-if-true
            w1727 = TRUE ("电动缸使能")
            n996 = local write "回零完成"(FALSE ("回零完成")) -> ()
            n997 = local write "测头机构轴使能"(w1727) -> ()
            n998 = local write "旋转齿条轴使能"(w1727) -> ()
            n999 = local write "电动缸使能"(w1727) -> ()
            n1000 = Wait Until Next ms Multiple(millisecond multiple=u32 50 ("毫秒倍数")) -> ()  [unwired: 1 out]
            n1001 = Greater Or Equal?(x=w1724, y=30) -> (x >= y?=w1722:bool)
          }
        }
      }
      n1002 = call "ADO Connection Create.vi"() -> ("error out"=w1720:errorcluster, "ADODB._Connection Out"=w1721:refnum<k7>)  [unwired: 10 in]
      n1003 = call "ADO Connection Open.vi"("error in (no error)"=w1720, "ConnectionString"="Provider=Microsoft.Jet.OLEDB.4.0;Data Source=D:\\Q14070-Z060人机界面\\参数\\参数Z060.mdb;Persist Security Info=False;Jet OLEDB:Database Password=123;", "ADODB._Connection In"=w1721) -> ("error out"=w1717:errorcluster, "ADODB._Connection Out"=w1719:refnum<k7>)  [unwired: 7 in]
    }
    frame #1 {
      n1004 = while {
        tunnel: w1729 -> [w1731]
        tunnel: w1728 -> [w1730]
        stop <- w1735 stop-if-true
        n1005 = Wait (ms)(milliseconds to wait=u32 50 ("等待时间（毫秒）")) -> ()  [unwired: 1 out]
        n1006 = First Call?() -> (First Call?: T/F=w1734:bool)
        n1007 = Or(x=w1734, y="参数加载") -> (x .or. y?=w1733:bool)
        n1008 = case shown="真" w1733 {
          tunnel: w1731 -> [_ w1738]
          tunnel: w1730 -> [_ w1737]
          frame False {
          }
          frame True {
            n1009 = stacked-sequence {
              tunnel: w1738 -> [w1744 w1755 w1813]
              tunnel: w1737 -> [w1739 _ _]
              frame #0 {
                n1010 = call "SQL Execute.vi"("error in (no error)"=w1739, "Command Text"="SELECT * FROM 测试参数表", "ADODB._Connection In"=w1744) -> ("Data"=w1742:string[][])  [unwired: 5 in, 3 out]
                n1011 = Index Array(array=w1742, index (col)=0 ("索引 (行)")) -> (element=w1746:string[])  [unwired: 1 in]
                n1012 = Array Size(array=w1746) -> (size(s)=w1741:i32)
                "型号数量" <- w1741
                n1013 = while {
                  shift-right: [w1753] -> w1745
                  shift-left: i32[] [] -> [w1752]
                  tunnel: w1741 -> [w1750]
                  i -> [w1751]
                  stop <- w1749 stop-if-true
                  n1014 = Greater Or Equal?(x=w1751, y=w1750) -> (x >= y?=w1749:bool)
                  n1015 = Build Array (concatenate)(w1752, w1751) -> (w1753:i32[])
                }
                n1016 = Build Cluster Array "索引与捆绑簇数组"(w1746, w1745) -> (w1740:cluster{"String":string, i32}[])
                n1017 = property on="型号选择" class="Ring (严格)"("StringsAndValues[]"=w1740) -> ()  [unwired: 2 in, 2 out]
              }
              frame #1 {
                n1018 = property on="型号选择" class="Ring (严格)"() -> ("RingText.Text"=w1756:string)  [unwired: 2 in, 2 out]
                n1019 = call "创建文本2"("型号选择"=w1756) -> ("Result"=w1760:string)  [unwired: 13 in, 1 out]
                n1020 = call "SQL Execute.vi"("Command Text"=w1760, "ADODB._Connection In"=w1755) -> ("Data"=w1759:string[][])  [unwired: 6 in, 3 out]
                n1021 = Index Array(array=w1759, index (row)=0 ("索引 (行)")) -> (element=w1757:string[])  [unwired: 1 in]
                n1022 = Fract/Exp String To Number ("分数/指数字符串至数值转换")(string=w1757) -> (number=w1754:dbl[])  [unwired: 3 in, 1 out]
                n1023 = stacked-sequence {
                  tunnel: w1754 -> [w1789]
                  frame #0 {
                    n1024 = Index Array ("索引数组")(array=w1789, index #1=2 ("索引"), index #2=3 ("索引"), index #3=4 ("索引"), index #4=5 ("索引"), index #5=6 ("索引"), index #6=7 ("索引"), index #7=8 ("索引"), index #8=9 ("索引"), index #9=10 ("索引"), index #10=11 ("索引"), index #11=12 ("索引"), index #12=13 ("索引"), index #13=14 ("索引"), index #14=15 ("索引"), index #15=16 ("索引"), index #16=17 ("索引"), index #17=18 ("索引"), index #18=19 ("索引"), index #19=20 ("索引")) -> (element #1=w1788:dbl, element #2=w1787:dbl, element #3=w1786:dbl, element #4=w1785:dbl, element #5=w1784:dbl, element #6=w1783:dbl, element #7=w1782:dbl, element #8=w1781:dbl, element #9=w1780:dbl, element #10=w1779:dbl, element #11=w1772:dbl, element #12=w1771:dbl, element #13=w1770:dbl, element #14=w1769:dbl, element #15=w1768:dbl, element #16=w1767:dbl, element #17=w1764:dbl, element #18=w1763:dbl, element #19=w1761:dbl)
                    n1025 = local write "测头机构轴移动速度"(w1788) -> ()
                    n1026 = local write "总圈数标准"(w1764) -> ()
                    n1027 = local write "总圈数最大值"(w1763) -> ()
                    n1028 = local write "平均轴向力标准(N) max"(w1767) -> ()
                    n1029 = local write "平均轴向力标准(N)"(w1768) -> ()
                    n1030 = local write "测头机构轴检测位"(w1787) -> ()
                    n1031 = local write "测头机构轴后退位"(w1785) -> ()
                    n1032 = local write "测头机构轴待检位"(w1786) -> ()
                    n1033 = local write "旋转齿条轴找帽转速"(w1781) -> ()
                    n1034 = local write "旋转齿条轴测量转速"(w1780) -> ()
                    n1035 = local write "转向器中心"(w1761) -> ()
                    n1036 = local write "总行程标准(mm)"(w1772) -> ()
                    n1037 = local write "最大轴向力标准(N)"(w1770) -> ()
                    n1038 = local write "齿条移动速度"(w1784) -> ()
                    n1039 = local write "齿条左极限"(w1783) -> ()
                    n1040 = local write "齿条右极限"(w1782) -> ()
                    n1041 = local write "力波动标准(N)"(w1769) -> ()
                    n1042 = local write "总行程最大值"(w1771) -> ()
                    n1043 = local write "测量点扭矩"(w1779) -> ()
                  }
                }
              }
              frame #2 {
                n1044 = call "SQL Execute.vi"("Command Text"="SELECT * FROM 传感器校验表 where ID='1'", "ADODB._Connection In"=w1813) -> ("Data"=w1815:string[][])  [unwired: 6 in, 3 out]
                n1045 = Index Array(array=w1815) -> (element=w1816:string[])  [unwired: 2 in]
                n1046 = Fract/Exp String To Number ("分数/指数字符串至数值转换")(string=w1816) -> (number=w1806:dbl[])  [unwired: 3 in, 1 out]
                n1047 = Index Array(array=w1806, index #1=1 ("索引"), index #2=2 ("索引"), index #3=3 ("索引"), index #4=4 ("索引"), index #5=5 ("索引"), index #6=6 ("索引")) -> (element #1=w1805:dbl, element #2=w1804:dbl, element #3=w1803:dbl, element #4=w1802:dbl, element #5=w1801:dbl, element #6=w1800:dbl)
                n1048 = local write "间隙位移零点偏移"(w1805) -> ()
                n1049 = local write "间隙位移比例偏移"(w1804) -> ()
                n1050 = local write "齿条推拉力零点偏移"(w1803) -> ()
                n1051 = local write "齿条推拉力比例偏移"(w1802) -> ()
                n1052 = local write "齿条扭矩零点偏移"(w1801) -> ()
                n1053 = local write "齿条扭矩比例偏移"(w1800) -> ()
              }
            }
          }
        }
        n1054 = local read "停止"() -> (w1735:bool)
        "ADODB._Connection Out 2" <- w1731
      }
    }
  }
  n1055 = while {
    stop <- w1818 stop-if-true
    n1056 = local read "rfid工步号"() -> (w1817:u32)
    n1057 = case shown="10" w1817 {
      frame 0, Default {
      }
      frame 10 {
        n1058 = flat-sequence {
          tunnel: [w1828] -> w1822
          tunnel: w1822 -> [w1830]
          tunnel: [w1829] -> w1821
          tunnel: w1821 -> [w1832]
          tunnel: [w1832] -> w1820
          tunnel: w1820 -> [w1835]
          frame #0 {
            n1059 = while {
              stop <- w1823 stop-if-true
              n1060 = local read "rfid触发"() -> (w1823:bool)
              n1061 = Wait Until Next ms Multiple(millisecond multiple=u32 50 ("毫秒倍数")) -> ()  [unwired: 1 out]
            }
          }
          frame #1 {
            n1062 = local write "芯片ID"("" ("随行板ID")) -> ()
            n1063 = local write "rfid完成"(FALSE ("RFID完成")) -> ()
            n1064 = local write "rfid触发"(FALSE ("RFID读取触发")) -> ()
          }
          frame #2 {
            n1065 = local read "Z060BRFID"() -> (w1828:string)
            n1066 = local write "芯片ID"(w1828) -> ()
          }
          frame #3 {
            n1067 = call "查询产品ID.vi"("芯片编码"=w1830) -> ("产品ID"=w1829:string)  [unwired: 8 in, 2 out]
            "读取产品ID" <- w1829
          }
          frame #4 {
            n1068 = Wait (ms)(milliseconds to wait=u32 500 ("等待时间（毫秒）")) -> ()  [unwired: 1 out]
          }
          frame #5 {
            n1069 = call "查询上序合格.vi"("产品ID"=w1835) -> ("本序已做"=w1833:bool, "上序合格"=w1834:bool)  [unwired: 8 in, 1 out]
            n1070 = Not(x=w1834) -> (.not. x?=w1836:bool)
            n1071 = local write "上序合格"(w1834) -> ()
            n1072 = local write "本序已做"(w1833) -> ()
            n1073 = local write "上序不合格"(w1836) -> ()
          }
          frame #6 {
            n1074 = local write "rfid完成"(TRUE ("RFID读取完成")) -> ()
            n1075 = Wait Until Next ms Multiple(millisecond multiple=u32 500 ("毫秒倍数")) -> ()  [unwired: 1 out]
          }
          frame #7 {
            "rfid工步号" <- 15.0 ("工步号")
          }
        }
      }
      frame 210 {
        n1076 = local read "读取产品ID"() -> (w1840:string)
        n1077 = local write "产品ID"(w1840) -> ()
      }
    }
    n1078 = Wait Until Next ms Multiple(millisecond multiple=u32 50 ("毫秒倍数")) -> ()  [unwired: 1 out]
    n1079 = local read "停止"() -> (w1818:bool)
  }
  n1080 = flat-sequence {
    tunnel: [w1841] -> w4
    tunnel: w4 -> [w1847]
    tunnel: [w1846] -> w3
    tunnel: w3 -> [w1913]
    frame #0 {
      n1081 = call "PCI1240U初始化.vi"() -> ("旋转电机"=→"旋转齿条电机":u32, "电动缸电机"=→"电动缸电机":u32, "DeviceHandle"=→"DeviceHandle":u32, "进给电机"=→"测头机构电机":u32)  [unwired: 6 in, 2 out]
      n1082 = call "PCI8622配置.vi"() -> ("DeviceID"=w1841:i32)  [unwired: 11 in]
    }
    frame #1 {
      n1083 = while {
        tunnel: w1847 -> [w1849]
        tunnel: [w1848] -> w1846
        stop <- "停止" stop-if-true
        n1084 = stacked-sequence {
          tunnel: w1849 -> [_ _ w1889]
          tunnel: [_ _ w1889] -> w1848
          frame #0 {
            n1085 = local read "测头机构电机"() -> (w1858:u32)
            n1086 = Boolean To (0,1)(Boolean="测头机构轴使能") -> (0, 1=w1856:i16)
            n1087 = call <userlib>:"Acm_AxSetSvOn.vi"("OnOff"=w1856, "AxisHandle"=w1858) -> ("AxisHandle"=w1855:u32)  [unwired: 1 in, 2 out]
            n1088 = call "PCI1220U进给轴速度设置.vi"("Change Velocity"="测头机构轴速度(mm/s)", "AxisHandle IN"=w1855) -> ("AxisHandle OUT"=w1853:u32)  [unwired: 9 in]
            n1089 = call "PCI1220U进给轴读取位置.vi"("AxisHandle IN"=w1853) -> ("位置"=→"测头机构轴位置(mm)":dbl)  [unwired: 9 in, 1 out]
          }
          frame #1 {
            n1090 = local read "电动缸电机"() -> (w1868:u32)
            n1091 = local read "旋转齿条电机"() -> (w1867:u32)
            n1092 = Boolean To (0,1)(Boolean="电动缸使能") -> (0, 1=w1872:i16)
            n1093 = Boolean To (0,1)(Boolean="旋转齿条轴使能") -> (0, 1=w1866:i16)
            n1094 = call <userlib>:"Acm_AxSetSvOn.vi"("OnOff"=w1866, "AxisHandle"=w1867) -> ("AxisHandle"=w1869:u32)  [unwired: 1 in, 2 out]
            n1095 = call <userlib>:"Acm_AxSetSvOn.vi"("OnOff"=w1872, "AxisHandle"=w1868) -> ("AxisHandle"=w1871:u32)  [unwired: 1 in, 2 out]
            n1096 = call "PCI1220U扭矩轴速度设置.vi"("Change Velocity"="旋转齿条轴速度(°/s)", "AxisHandle IN"=w1869) -> ("AxisHandle OUT"=w1870:u32)  [unwired: 9 in]
            n1097 = call "PCI1240电动缸速度设置.vi"("Change Velocity"="电动缸速度(mm/s)", "AxisHandle IN"=w1871) -> ("AxisHandle OUT"=w1859:u32)  [unwired: 9 in]
            n1098 = call "PCI1220U扭矩轴读取位置.vi"("AxisHandle IN"=w1870) -> ("位置"=→"旋转齿条轴位置(°)":dbl)  [unwired: 9 in, 1 out]
            n1099 = call "PCI1240电动缸读取位置.vi"("AxisHandle IN"=w1859) -> ("位置"=→"电动缸位置(mm)":dbl)  [unwired: 9 in, 1 out]
          }
          frame #2 {
            w1905 = 0  # nRetSizeWords
            w1906 = 2048  # nReadSizeWords
            # "hDevice"
            n1100 = Initialize Array(u16 0, 2048 ("dimension size")) -> (w1896:u16[])
            n1101 = dll-call lib="PCI8622_32.dll" fn="PCI8622_ReadDeviceProAD_Npt" label="ReadDeviceProAD_Npt"("hDevice"=w1889, "ADBuffer[]"=w1896, "nReadSizeWords"=w1906, "nRetSizeWords"=w1905) -> ("ADBuffer[]"=w1899:u16[])  [unwired: 7 in, 2 out]
            n1102 = Divide(x=w1899, y=65536.01) -> (x/y=w1900:dbl[])
            n1103 = Multiply(x=w1900, y=20) -> (x*y=w1903:dbl[])
            n1104 = Subtract(x=w1903, y=10) -> (x-y=w1895:dbl[])
            n1105 = Decimate 1D Array ("抽取一维数组")(w1895) -> (w1883:dbl[], w1884:dbl[], w1882:dbl[])  [unwired: 5 out]
            n1106 = Add Array Elements(numeric array=w1883) -> (sum=w1892:dbl)
            n1107 = Add Array Elements(numeric array=w1882) -> (sum=w1893:dbl)
            n1108 = Array Size(array=w1883) -> (size(s)=w1891:i32)
            n1109 = Add Array Elements(numeric array=w1884) -> (sum=w1888:dbl)
            n1110 = Array Size(array=w1882) -> (size(s)=w1894:i32)
            n1111 = Array Size(array=w1884) -> (size(s)=w1890:i32)
            n1112 = Divide(x=w1892, y=w1891) -> (x/y=w1881:dbl)
            n1113 = Divide(x=w1893, y=w1894) -> (x/y=w1875:dbl)
            n1114 = Divide(x=w1888, y=w1890) -> (x/y=w1878:dbl)
            n1115 = Subtract(x=w1875, y=4.43) -> (x-y=w1873:dbl)
            n1116 = Multiply(x=w1881, y=2.0) -> (x*y=w1876:dbl)
            n1117 = Multiply(x=w1878, y=200.0) -> (x*y=w1877:dbl)
            n1118 = local read "间隙位移比例偏移"() -> (w1910:dbl)
            n1119 = local read "间隙位移零点偏移"() -> (w1909:dbl)
            n1120 = local read "齿条扭矩零点偏移"() -> (w1911:dbl)
            n1121 = local read "齿条扭矩比例偏移"() -> (w1912:dbl)
            n1122 = local read "齿条推拉力比例偏移"() -> (w1908:dbl)
            n1123 = local read "齿条推拉力零点偏移"() -> (w1907:dbl)
            n1124 = call "传感器校订.vi"("零点"=w1911, "比例"=w1912, "传感器"=w1876) -> ("示值"=→"齿条扭矩(Nm)":dbl)  [unwired: 8 in]
            n1125 = call "传感器校订.vi"("零点"=w1909, "比例"=w1910, "传感器"=w1873) -> ("示值"=→"间隙位移(mm)":dbl)  [unwired: 8 in]
            n1126 = call "传感器校订.vi"("零点"=w1907, "比例"=w1908, "传感器"=w1877) -> ("示值"=→"齿条推拉力(N)":dbl)  [unwired: 8 in]
          }
        }
        n1127 = Wait Until Next ms Multiple(millisecond multiple=u32 50 ("毫秒倍数")) -> ()  [unwired: 1 out]
      }
    }
    frame #2 {
      n1128 = dll-call lib="PCI8622_32.dll" fn="PCI8622_StopDeviceProAD" label="StopDeviceProAD"("hDevice"=w1913) -> ("hDevice"=w1914:i32)  [unwired: 4 in, 2 out]
      n1129 = dll-call lib="PCI8622_32.dll" fn="PCI8622_ReleaseDeviceProAD" label="ReleaseDeviceProAD"("hDevice"=w1914) -> ()  [unwired: 5 in, 2 out]
      n1130 = dll-call lib="PCI8622_32.dll" fn="PCI8622_ReleaseDevice" label="ReleaseDevice"("hDevice"=w1913) -> ()  [unwired: 5 in, 2 out]
    }
  }
